vi "TweezerTron.vi"() -> ()   [LabVIEW 2020]
uses:
  _Controls/PIFOC Position.ctl
  _Controls/Confocal Controls.ctl
  _Controls/iFlex.ctl
  _Controls/Manlight Controls.ctl
  _Controls/Exp Params.ctl
  _Controls/Image Thresholds.ctl
  _Controls/Spots.ctl
  _Controls/Tweezertron Ctrl Refs.ctl
  _Controls/Review Ctrl Refs.ctl
  _Controls/Timer actions.ctl
  <vilib>/Platform/TimedLoop/XDataNode/timing_clust.ctl
  <vilib>/Platform/TimedLoop/XDataNode/nitl_modes.ctl
  <vilib>/Platform/TimedLoop/XDataNode/wakeup.ctl
  _Controls/Logging Queue Cluster.ctl
  _Globals/Global Controls.vi
  Instruments/Physik Instrumente/SDK/GCS_LabVIEW_digital/Low Level/Communication.llb/Global1.vi
  <vilib>/Platform/TimedLoop/XDataNode/XDataNode.xnode
  Instruments/Thorlabs/ECU_SDK/ThorECU.lvlib
  Instruments/Thorlabs/LSM_SDK/ThorConfocal.lvlib
  Instruments/Thorlabs/MPH_SDK/MPH16.lvlib
  <vilib>/Platform/TimedLoop/XDataNode/XDNodeRunTimeDep.lvlib
panel:
  out "pane closed":bool
  out "Pause Live Imaging":bool
  out "Live Imaging":bool
  out "Live Review":bool
  out "LiveDisp":T1(plugin-control)
  in  "Control Tabs":T2(tab)
  in  "img thresholds":T3={"Channel A"={1, 16382}, "Channel B"={1, 16382}} {"Channel B" scale=0.0..16382.0; "Channel A" scale=0.0..16382.0}
  in  "Manlight Controls":T4 caption="Trapping Laser" {"Manlight Power" min=0.0 max=10.0 step=0.1 scale=0.0..10.0}
  in  "Stop Live Imaging":bool
  in  "Start Live Imaging":bool
  in  "LSM Settings":T5={"Channel Selection"=enum."A", "Pixel Count"={"Pixels in X"=512, "Pixels in Y"=512}, "Field Size"=90.0, "Frames"=2, "Averaging"=FALSE, "Alignment"=0.0, "Scan Mode"=TRUE, "Gain"={"Gain A"=1, "Gain B"=1}, "Enable PMTs"={"A"=TRUE, "B"=TRUE}, "Voltage Range"={"Range A"=10, "Range B"=10}, "Multi Frame Count"=0.0, "Trigger Mode"=2.0, "Real Time Averaging"=TRUE, "PFOV"=0.0, "MicronsPerPx"=0.0} caption="Confocal Scanner" {"Field Size" min=5.0 max=255.0 step=1.0 scale=5.0..255.0; "PFOV" min=1.0 max=300.0 step=0.1; "MicronsPerPx" min=0.01 step=0.01 format="%.2f"; "Gain"."Gain B" min=1 max=100 step=1; "Gain"."Gain A" min=1 max=100 step=1; "Voltage Range"."Range B" items=["100mV"=5, "200mV"=6, "400mV"=7, "1V"=10, "2V"=11, "4V"=12]; "Voltage Range"."Range A" items=["100mV"=5, "200mV"=6, "400mV"=7, "1V"=10, "2V"=11, "4V"=12]; "Pixel Count"."Pixels in Y" items=["32"=32, "64"=64, "128"=128, "256"=256, "512"=512, "1024"=1024, "2048"=2048]; "Pixel Count"."Pixels in X" items=["32"=32, "64"=64, "128"=128, "256"=256, "512"=512, "1024"=1024, "2048"=2048]}
  in  "PIFOC Settings":T6={"PIFOC Position (mm) [SET]"=0.0, "PIFOC Position\n(um) [ACT]"=0.0087, "last command"=""} {"PIFOC Position\n(um) [ACT]" format="%.2f"; "PIFOC Position (mm) [SET]" min=0.0 max=100.0 step=0.1 scale=0.0..100.0}
  out "LSM Frame Rate":dbl=15.255953524835265 caption="Frame Rate (Hz)" format="%#.0f"
  in  "iFlex Control":T7 caption="Confocal Laser" {"561" min=12.5 max=100.0 step=0.1 scale=0.0..100.0; "488" min=30.0 max=100.0 step=0.1 scale=0.0..100.0}
  in  "PinSelector":dbl(ring)=6.0 caption="Pin Hole (mm)" items=["25", "30", "35", "40", "45", "50", "60", "70", "80", "90", "100", "125", "200", "300", "1000", "2000"]
  in  "Spots":T8=[{"Intensity"=1.0, "Vortex"=0.0, "Phase"=0.0, "X"=7.0, "Y"=0.0, "Z"=0.0}] {"Z" format="%_4g"; "Y" format="%_4g"; "X" format="%_4g"; "Phase" format="%_4g"; "Intensity" format="%_4g"}
  out "Saving To Disk":i32(slide) scale=0.0..8000.0
  out "Acquiring Data":i32(slide) max=1000 scale=0.0..8000.0
  in  "Stop Experiment":bool
  in  "Exp Params":T9={"Experiment Type"="2D Snapshot", "Experiment Name"="Experiment_1", "ExpPath"=path "E:/Data", "TSFrames"=1000, "TSfps"=1000, "ZTSFrames"=1000, "ZTSdt"=1, "Streaming"=FALSE, "Z Stack Settings"={"Start"=0.0, "Step Size"=0.1, "Finish"=1.0}, "total images"=1, "tdms ref"=refnum, "frame #"=0, "images per stack"=1, "total stacks"=1, "period"=1, "PI MVR Increment"=""} {"period" min=1; "total stacks" min=1; "images per stack" min=1; "total images" min=1; "Z Stack Settings"."Start" min=0.0 max=100.0 step=0.1; "Z Stack Settings"."Step Size" min=0.1 max=100.0 step=0.1; "Z Stack Settings"."Finish" min=0.0 max=100.0 step=0.1; "TSFrames" min=1 step=1; "ZTSdt" min=1 step=1; "ZTSFrames" min=2 step=1; "TSfps" min=1 max=1000 step=1}
  in  "Start Experiment":bool
  out "#stack":i32 caption="Stacks"
  in  "Rev Path":path=path "D:/Data/test/qwerty6/qwerty6.tdms" caption="Path to Experiment TDMS File"
  out "dts (ms)":u64[](graph)
  in  "RevFrame":i32(slide)=1 caption="Frame" min=1 max=8001 step=1 scale=0.9..8001.0
  out "Time (s)":dbl
  out "Position (um)":dbl=49.99
  out "dt (ms)":u32
  in  "End Review":bool
  out "PIFOC Positions":cluster{dbl[], "PI pos (um)":dbl[]}(graph)
  in  "Review Experiment":bool
  in  "Save TIFFs":bool
  out "Exporting TIFFS":i32(slide) max=1000 scale=0.0..8000.0
  out "status":string="Status"
  in  "Master Stop":bool
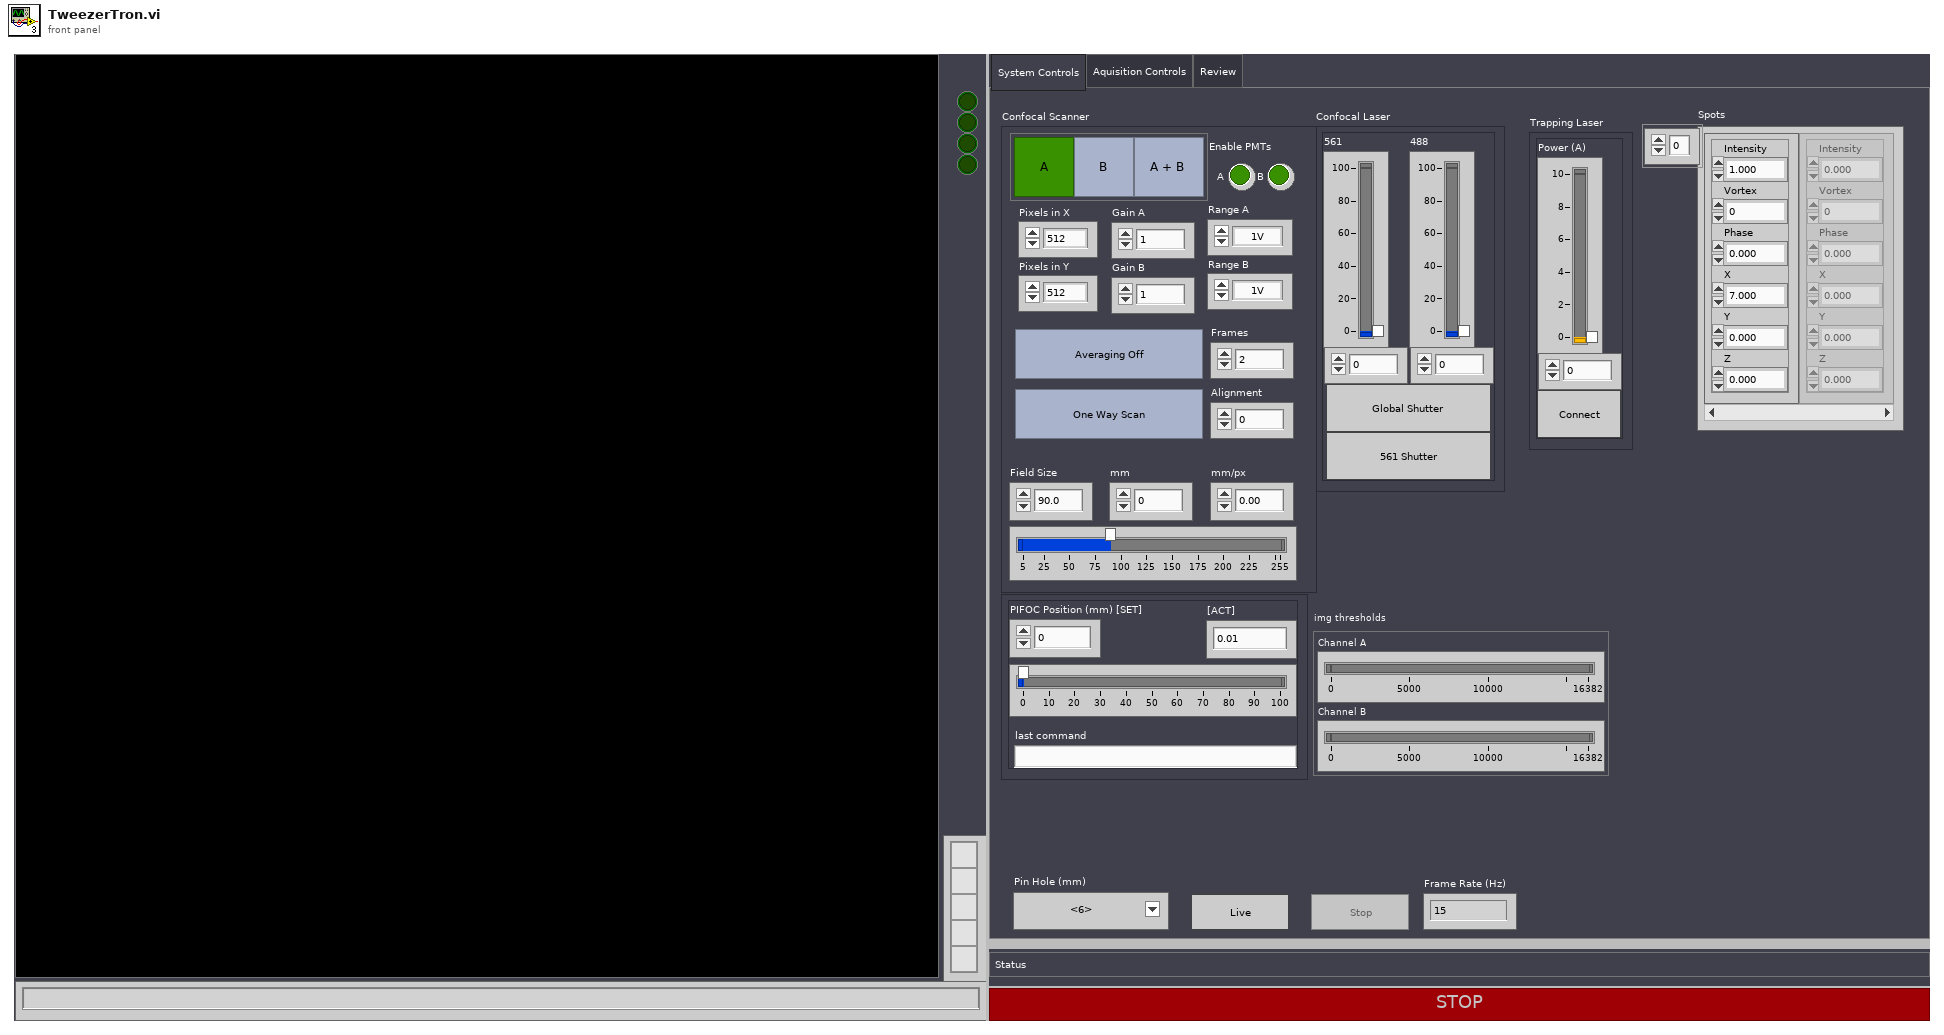
[diagram p1: front panel]
types:
  T1 = typedef "IMAQ Image.ctl" = refnum<image>
  T2 = enum32{"System Controls", "Aquisition Controls", "Review"}
  T3 = typedef "Image Thresholds.ctl" = cluster{"Channel A":cluster{u16, u16}, "Channel B":cluster{u16, u16}}
  T4 = typedef "Manlight Controls.ctl" = cluster{"Manlight Power":dbl, "Open Serial":bool, "VISA Refnum":refnum<visa-resource-name>}
  T5 = typedef "Confocal Controls.ctl" = cluster{"Channel Selection":enum32{"A", "B", "AB"}, "Pixel Count":cluster{"Pixels in X":u32, "Pixels in Y":u32}, "Field Size":dbl, "Frames":u8, "Averaging":bool, "Alignment":dbl, "Scan Mode":bool, "Gain":cluster{"Gain A":u8, "Gain B":u8}, "Enable PMTs":cluster{"A":bool, "B":bool}, "Voltage Range":cluster{"Range A":u16, "Range B":u16}, "Multi Frame Count":dbl, "Trigger Mode":dbl, "Real Time Averaging":bool, "PFOV":dbl, "MicronsPerPx":dbl}
  T6 = typedef "PIFOC Position.ctl" = cluster{"PIFOC Position (mm) [SET]":dbl, "PIFOC Position\n(um) [ACT]":dbl, "last command":string}
  T7 = typedef "iFlex.ctl" = cluster{"561":dbl, "488":dbl, "Global Shutter":bool, "561 Shutter":bool}
  T8 = typedef "Spots.ctl" = cluster{"Intensity":dbl, "Vortex":dbl, "Phase":dbl, "X":dbl, "Y":dbl, "Z":dbl}[]
  T9 = typedef "Exp Params.ctl" = cluster{"Experiment Type":string, "Experiment Name":string, "ExpPath":path, "TSFrames":i32, "TSfps":i32, "ZTSFrames":i32, "ZTSdt":i32, "Streaming":bool, "Z Stack Settings":cluster{"Start":dbl, "Step Size":dbl, "Finish":dbl}, "total images":i32, "tdms ref":refnum<k34>, "frame #":i64, "images per stack":i32, "total stacks":i32, "period":i32, "PI MVR Increment":string}
  T10 = typedef "Image Type" = u32
  T11 = typedef "Review Ctrl Refs.ctl" = cluster{"RevFrame":refnum<vi>, "dts (ms)":refnum<vi>, "PIFOC Positions":refnum<vi>}
  T12 = enum8{"Enabled", "Disabled", "Disabled and Grayed Out"}
  T13 = typedef "Tweezertron Ctrl Refs.ctl" = cluster{"LSM Settings":refnum<vi>, "iFlex Control":refnum<vi>, "PIFOC Settings":refnum<vi>, "PinSelector":refnum<vi>, "Manlight Controls":refnum<vi>, "Exp Params":refnum<vi>, "Image Thresholds":refnum<vi>, "RevFrame":refnum<vi>, "Spots":refnum<vi>}
  T14 = cluster{"Confocal":bool, "Pinhole":bool, "PIFOC":bool, "Manlight":bool, "iFlex":bool, "SLM":bool}
  T15 = typedef "All Controls For Saving.ctl" = cluster{"Confocal Controls":T5, "iFlex Control":T7, "PIFOC Settings":T6, "PinSelector":dbl, "Manlight Controls":T4, "Exp Params":T9, "Spots":T8}
  T16 = typedef "Notifiers.ctl" = cluster{"Instrument Control":refnum<notifier>, "LSM Run Live":refnum<notifier>, "LSM Run Exp":refnum<notifier>, "Review Exp":refnum<notifier>}
  T17 = typedef "Timer actions.ctl" = enum16{"Reset", "Snap", "Total"}
  T18 = cluster{"notification":string, "Variant":variant}
  T19 = cluster{"561":bool, "488":bool, "Global Shutter":bool, "561 Shutter":bool}
  T20 = cluster{"New LSM Settings":T5, "index of change":i32}
  T21 = cluster{"iFlex Controls":T7, "appended array":i32[]}
  T22 = cluster{"Experiment Type":string, "Variant":variant}
  T23 = typedef "XDNodeRunTimeDep.lvlib/timing_clust.ctl" = cluster{"Expected End [f-1]":u64, "Actual End [f-1]":u64, "Finished Late? [f-1]":bool, "Expected End [i-1]":u64, "Actual End [i-1]":u64, "Finished Late? [i-1]":bool, "Expected Start [i]":u64, "Actual Start [i]":u64, "Expected Start [f]":u64, "Actual Start [f]":u64, "Source Name":string, "Structure Name":string, "Period":i64, "Deadline":i64, "Offset":i64, "Start":i64, "Priority":i32, "Timeout":i32, "Mode":T24, "Wakeup Reason":T25, "Error":errorcluster, "Source Type":string, "Secondary Source Type":string, "Global End Time":u64, "Global Start Time":u64, "Frame Duration":u64, "Iteration Duration":u64, "Assigned CPU":i32, "I/O Scan Engine Mode":u32}
  T24 = typedef "XDNodeRunTimeDep.lvlib/nitl_modes.ctl" = enum32{"No Change", "Process missed periods, maintain original phase", "Discard missed periods, maintain original phase", "Process missed periods, ignore original phase", "Discard missed periods, ignore original phase"}
  T25 = typedef "XDNodeRunTimeDep.lvlib/wakeup.ctl" = enum32{"Normal", "Aborted", "Asynchronous wakeup", "Timing source error", "Timed loop error", "Timeout"}
  T26 = typedef "Logging Queue Cluster.ctl" = cluster{"message":string, "Data for Logging":cluster{"pDataBuffer":u16[], "timestamp (ns)":u64, "PI pos (um)":dbl}, "Tweezertron Ctrl Refs":T13}
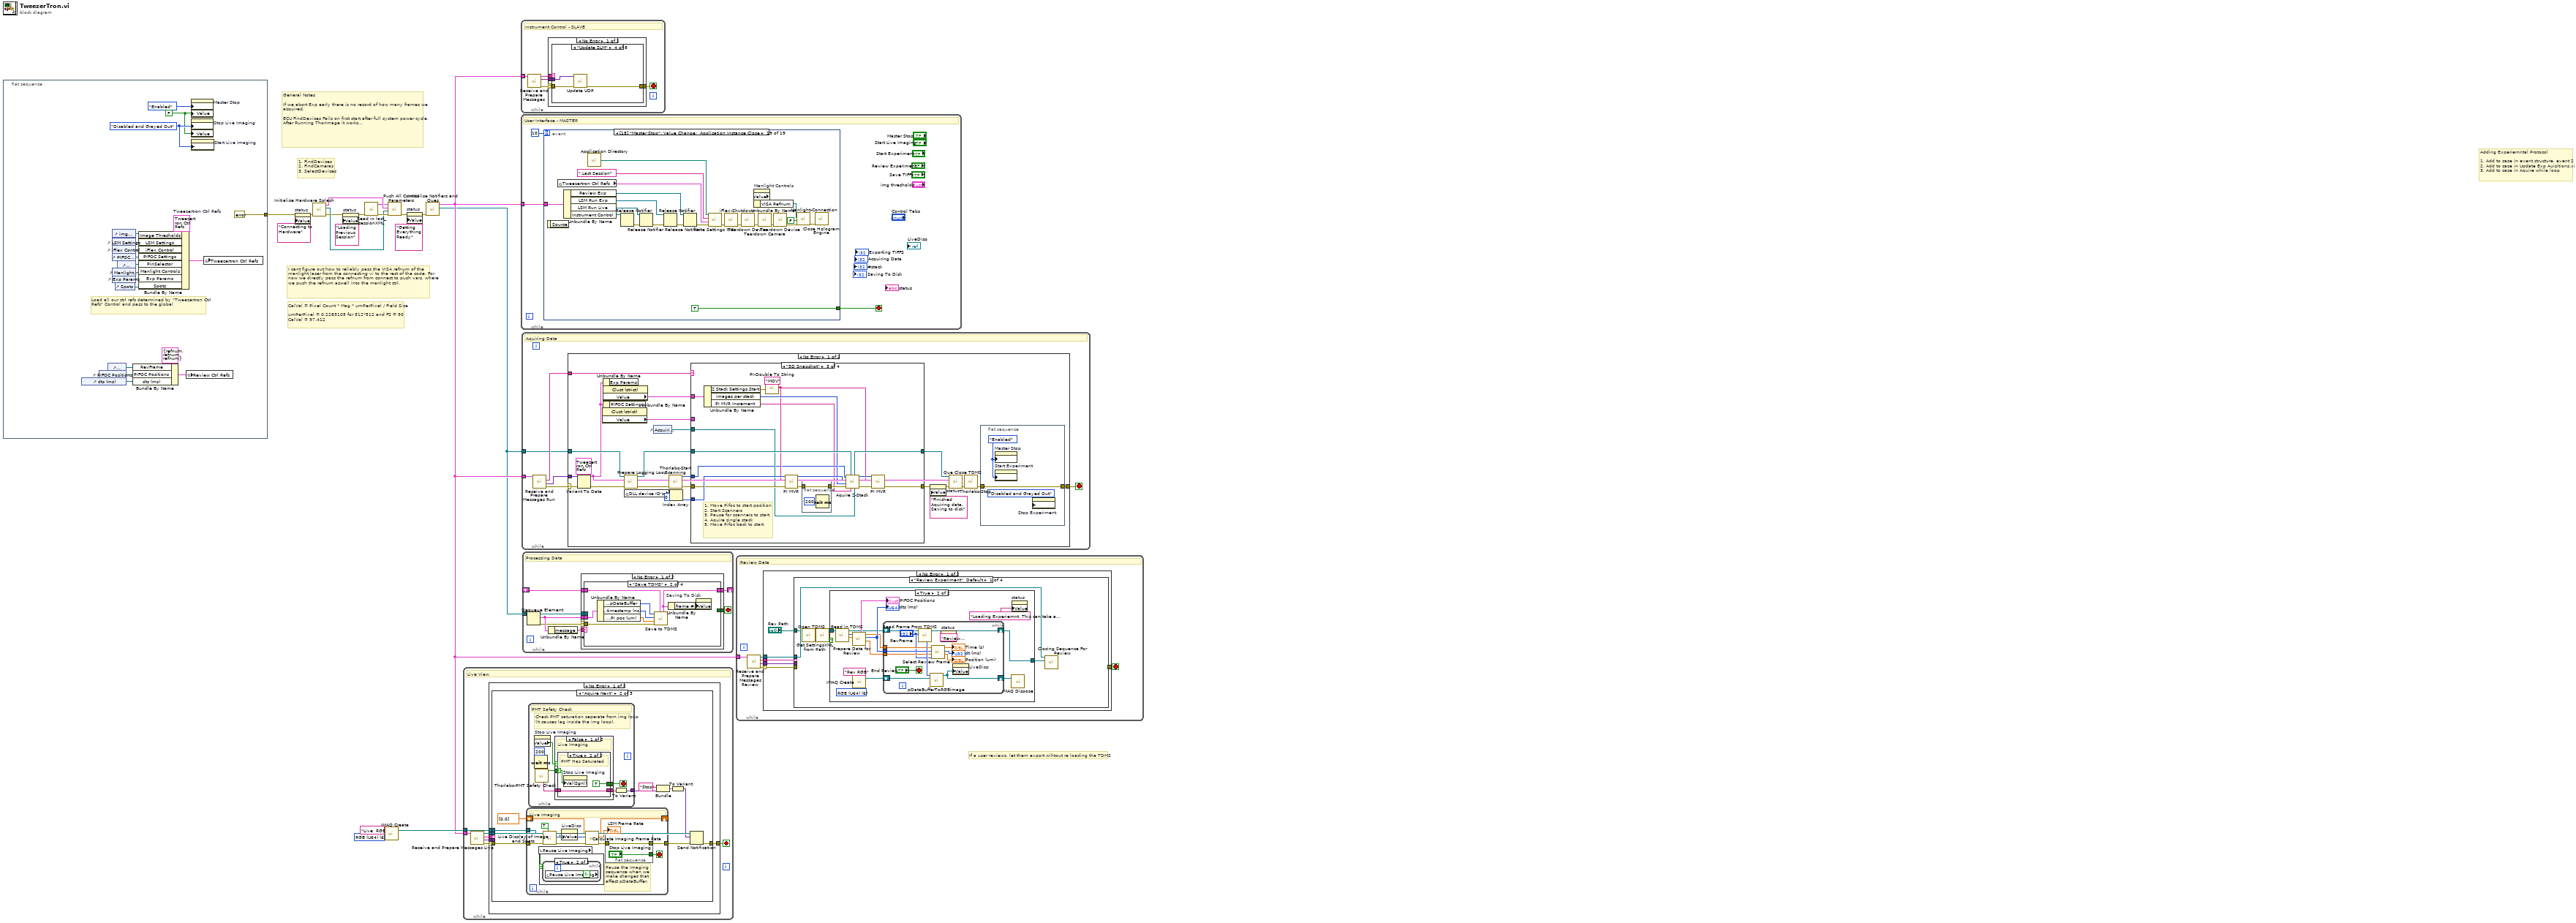
[diagram p0: block diagram]
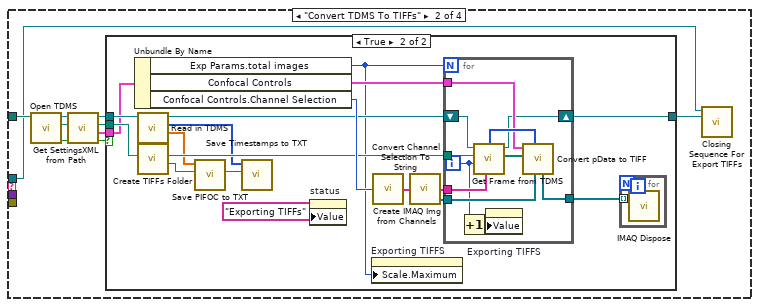
[diagram p3: hidden frame]
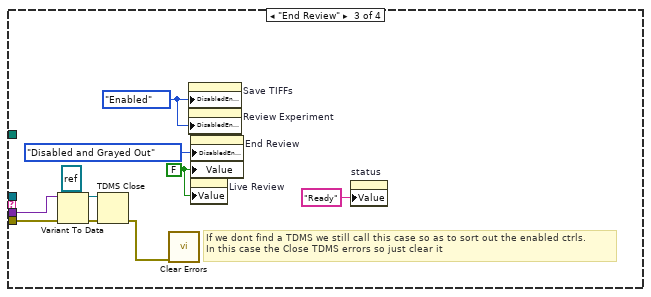
[diagram p5: hidden frame]
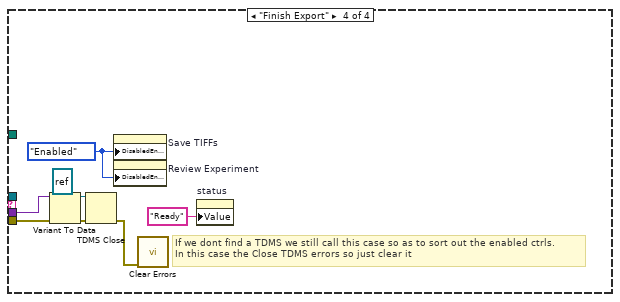
[diagram p6: hidden frame]
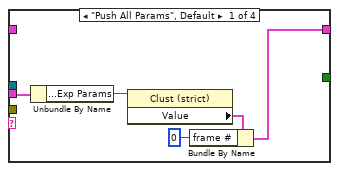
[diagram p8: hidden frame]
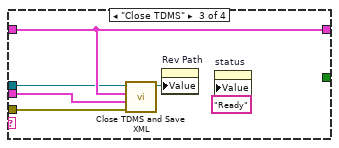
[diagram p9: hidden frame]
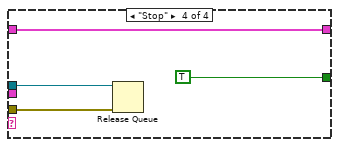
[diagram p10: hidden frame]
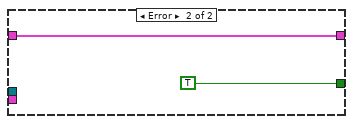
[diagram p11: hidden frame]
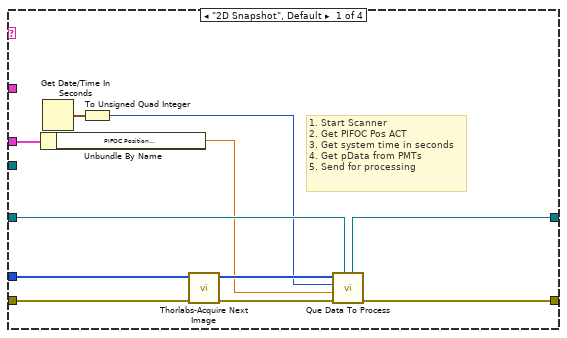
[diagram p12: hidden frame]
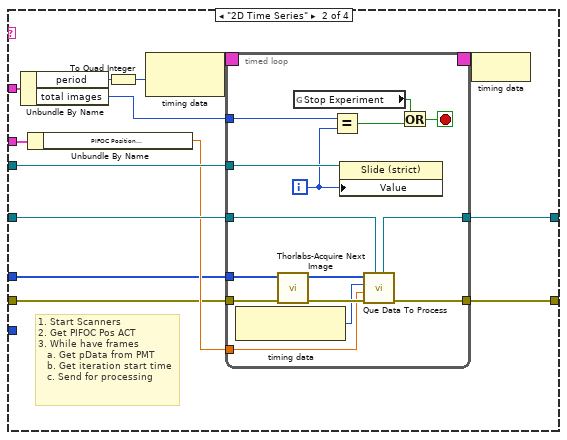
[diagram p13: hidden frame]
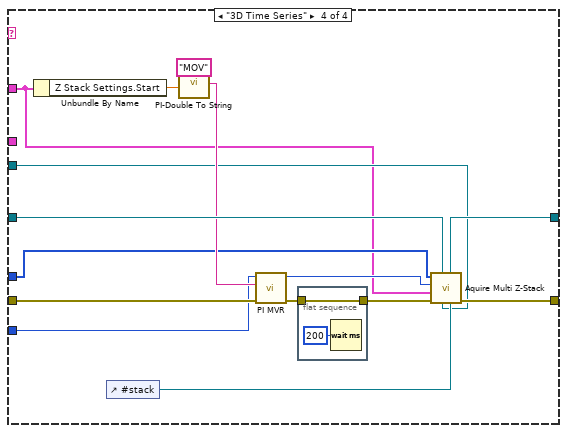
[diagram p14: hidden frame]
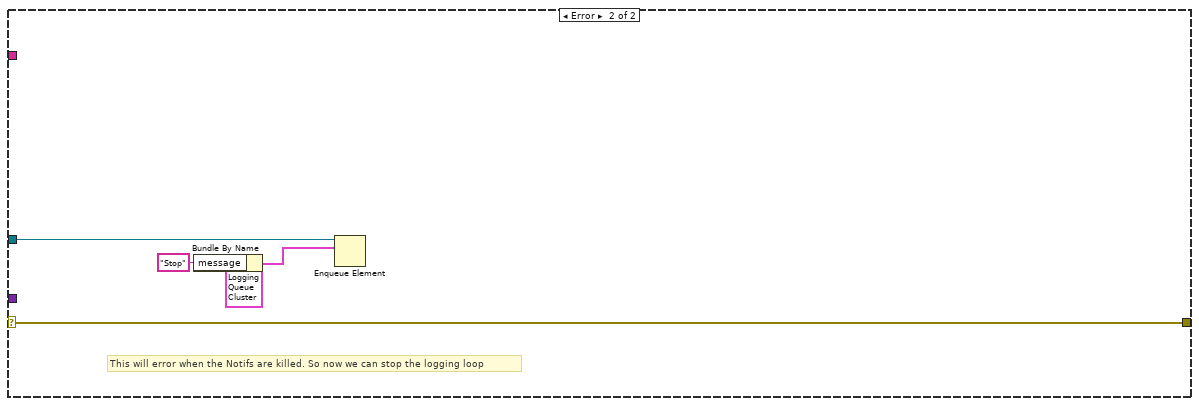
[diagram p15: hidden frame]
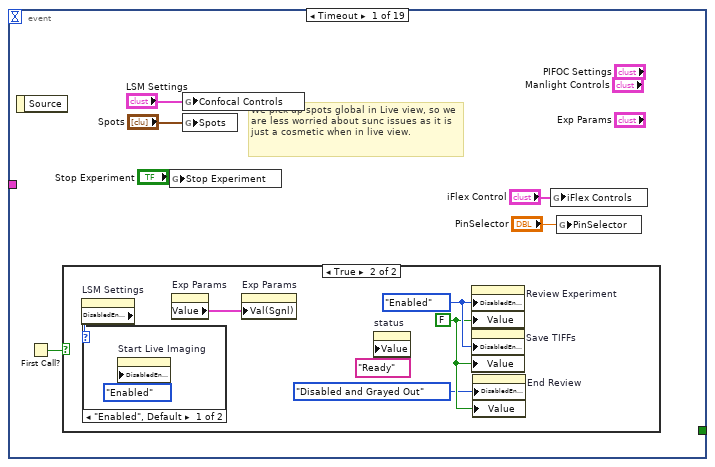
[diagram p16: hidden frame]
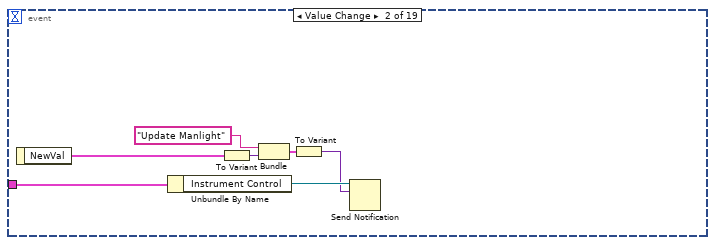
[diagram p19: hidden frame]
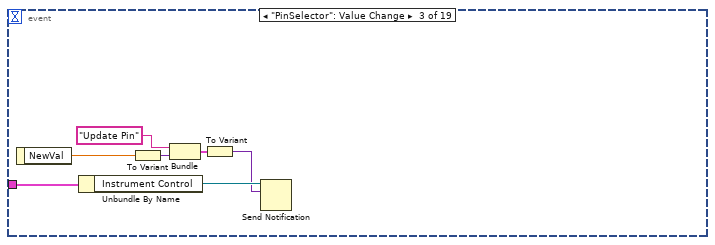
[diagram p20: hidden frame]
diagram:
  w15 = T10 6 items=["Grayscale (U8)", "Grayscale (I16)", "Grayscale (SGL)", "Complex (CSG)", "RGB (U32)", "HSL (U32)", "RGB (U64)", "Grayscale (U16)"] ("Image Type")
  # "If a user reviews, let them export wihtout re loading the TDMS"
  # "General Notes\n\nIf we abort Exp early there is no record of how many frames we acquired.\n\nECU FindDevices Fails on first start after full system power cycle. After Running ThorImage it works..."
  # "Adding Experiemntal Protocol\n\n1. Add to case in event structure, event 2\n2. Add to case in Update Exp Auisitions.vi\n3. Add to case in Aquire while loop"
  # "I cant figure out how to reliably pass the VISA refnum of the manlight laser from the connecting vi to the rest of the code. For now we directly pass the refnum from connect to push vars, where we push the refnum aswell into the manlight ctrl."
  # "CalVal = Pixel Count * Mag * umPerPixel / Field Size\n\numPerPixel = 0.2283105 for 512*512 and FS = 90\nCalVal = 97.412"
  # "1. FindDevices\n2. FindCameras\n3. SelectDevices"
  n1 = flat-sequence {
    tunnel: [errorcluster {"status"=FALSE, "code"=0, "source"=""} ("error constant")] -> w12
    frame #0 {
      w26 = FALSE ("Master Stop")
      w30 = T13 {"LSM Settings"=refnum, "iFlex Control"=refnum, "PIFOC Settings"=refnum, "PinSelector"=refnum, "Manlight Controls"=refnum, "Exp Params"=refnum, "Image Thresholds"=refnum, "RevFrame"=refnum, "Spots"=refnum}  # Tweezertron Ctrl Refs
      w28 = T12."Disabled and Grayed Out" ("Disabled")
      # "Load all our ctrl refs determined by \"Tweezertron Ctrl Refs\" Control and pass to the global"
      n2 = control-ref of="dts (ms)"() -> (w22:refnum<vi>)
      n3 = control-ref of="PIFOC Positions"() -> (w19:refnum<vi>)
      n4 = control-ref of="RevFrame"() -> (w23:refnum<vi>)
      n5 = control-ref of="img thresholds"() -> (w25:refnum<vi>)
      n6 = control-ref of="LSM Settings"() -> (w31:refnum<vi>)
      n7 = control-ref of="iFlex Control"() -> (w35:refnum<vi>)
      n8 = control-ref of="PIFOC Settings"() -> (w34:refnum<vi>)
      n9 = control-ref of="Manlight Controls"() -> (w29:refnum<vi>)
      n10 = control-ref of="Exp Params"() -> (w27:refnum<vi>)
      n11 = control-ref of="Spots"() -> (w20:refnum<vi>)
      n12 = control-ref of="PinSelector"() -> (w32:refnum<vi>)
      n13 = Bundle By Name(cluster=T11 {"RevFrame"=refnum, "dts (ms)"=refnum, "PIFOC Positions"=refnum} ("Review Ctrl Refs"), "RevFrame"=w23, "PIFOC Positions"=w19, "dts (ms)"=w22) -> (w21:T11)
      n14 = Bundle By Name(cluster=w30, "Image Thresholds"=w25, "LSM Settings"=w31, "iFlex Control"=w35, "PIFOC Settings"=w34, "PinSelector"=w32, "Manlight Controls"=w29, "Exp Params"=w27, "Spots"=w20) -> (w33:T13)
      n15 = global write "Global Controls.vi" "Review Ctrl Refs"(w21) -> ()
      n16 = property on="Master Stop" class="Bool (strict)"("DisabledEnum"=T12."Enabled" ("Disabled"), "Value"=w26) -> ()  [unwired: 2 in, 2 out]
      n17 = property on="Stop Live Imaging" class="Bool (strict)"("DisabledEnum"=w28, "Value"=w26) -> ()  [unwired: 2 in, 2 out]
      n18 = property on="Start Live Imaging" class="Bool"("DisabledEnum"=w28) -> ()  [unwired: 2 in, 2 out]
      n19 = global write "Global Controls.vi" "Tweezertron Ctrl Refs"(w33) -> ()
    }
  }
  n20 = property on="status" class="Str"(error in=w12, "Value"="Connecting to Hardware" ("status")) -> (error out=w17:errorcluster)  [unwired: 1 in, 1 out]
  n21 = call "Initialise Hardware Splash.vi"("error in (no error)"=w17) -> ("error out"=w1:errorcluster, "VISA Refnum out"=w5:refnum<visa-resource-name>, "Enabled Hardware"=w11:T14)  [unwired: 8 in]
  n22 = property on="status" class="Str"(error in=w1, "Value"="Loading Previous Session" ("status")) -> (error out=w14:errorcluster)  [unwired: 1 in, 1 out]
  n23 = call "Read in last_sessionXML.vi"("error in"=w14) -> ("error out"=w8:errorcluster, "All Controlls For Saving"=w9:T15)  [unwired: 9 in]
  n24 = call "IMAQ Create"("Image Name"="Live  RGB", "Image Type"=w15) -> ("New Image"=w4:T1)  [unwired: 3 in, 1 out]
  n25 = call "Push All Control Parameters.vi"("error in"=w8, "Manlight VISA Refnum"=w5, "Enabled Hardware"=w11, "All Controlls For Savinge"=w9) -> ("error out"=w6:errorcluster)  [unwired: 5 in]
  n26 = property on="status" class="Str"(error in=w6, "Value"="Getting Everything Ready" ("status")) -> (error out=w10:errorcluster)  [unwired: 1 in, 1 out]
  n27 = call "Initialise Notifiers and Ques.vi"("error in (no error)"=w10) -> ("Logging Queue out"=w2:refnum<queue>, "Notifiers"=w3:T16)  [unwired: 8 in, 1 out]
  n28 = while {
    tunnel: w4 -> [w44]
    tunnel: w3 -> [w38]
    stop <- w41 stop-if-true
    # "Live View"
    n29 = call "Receive and Prepare Messages Live.vi"("Notifiers"=w38) -> ("error out"=w42:errorcluster, "params"=w39:variant, "message"=w40:string, "LSM Run Live"=w43:refnum<notifier>)  [unwired: 6 in]
    n30 = case shown="No Error" w42 {
      selector: w42 -> [w49 w117]
      tunnel: w40 -> [w50 _]
      tunnel: w43 -> [w48 _]
      tunnel: w44 -> [w47 _]
      tunnel: [w46 w117] -> w41
      tunnel: w39 -> [w45 _]
      frame No Error {
        n31 = case shown="\"Aquire Next\"" w50 {
          tunnel: w49 -> [w61 w62 w115]
          tunnel: w48 -> [w55 w69 _]
          tunnel: w47 -> [_ w71 _]
          tunnel: [w54 w67 w114] -> w46
          tunnel: w45 -> [w53 _ w112]
          frame "Start" {
            n32 = global read "Global Controls.vi" "Tweezertron Ctrl Refs"() -> (w51:T13)
            n33 = Bundle("notification"="Aquire Next", "params"=w53) -> (w57:cluster{"notification":string, "params":variant})  [unwired: 1 in]
            n34 = call "Thorlabs-Start Scanning.vi"("error in (no error)"=w61, "Tweezertron Ctrl Refs"=w51) -> ("error out"=w60:errorcluster)  [unwired: 7 in, 2 out]
            n35 = To Variant(anything=w57) -> (Variant=w56:variant)
            n36 = Send Notification(notification=w56, notifier=w55, error in (no error)=w60) -> (error out=w59:errorcluster)  [unwired: 1 out]
            n37 = call "Get Kernel Time.vi"("error in (no error) in"=w59, "Action (Snap)"=Timer_actions."Reset") -> ("error out"=w54:errorcluster)  [unwired: 8 in, 1 out]
          }
          frame "Aquire Next" {
            n38 = while {
              tunnel: w71 -> [w97]
              tunnel: w62 -> [w102]
              tunnel: [w93] -> w70
              shift-right: [w101] -> _
              shift-left: dbl[] [0.0] -> [w95]
              stop <- w92 stop-if-true
              # "Pause the Imaging sequence when we make changes that affect pDataBuffer."
              # "Live Imaging"
              n39 = local read "Pause Live Imaging"() -> (w96:bool)
              n40 = case shown="True" w96 {
                frame False {
                }
                frame True {
                  n41 = while {
                    stop <- w105 continue-if-true
                    n42 = local read "Pause Live Imaging"() -> (w105:bool)
                  }
                }
              }
              n43 = call "Live Display of Image and Spots.vi"("Draw spots"=TRUE, "error in (no error)"=w102, "img dst"=w97) -> ("error out"=w98:errorcluster, "Frame Duration"=w100:i64, "img out"=w91:refnum<image>)  [unwired: 6 in]
              n44 = property on="LiveDisp" class="ImageControl"("Value"=w91) -> ()  [unwired: 2 in, 2 out]
              n45 = call "Calculate Imaging Frame Rate.vi"("error in (no error)"=w98, "Frame Duration"=w100, "Durations IN"=w95) -> ("error out"=w94:errorcluster, "LSM Frame Rate"=→"LSM Frame Rate":dbl, "Durations OUT"=w101:dbl[])  [unwired: 6 in]
              n46 = flat-sequence {
                tunnel: w94 -> [w104]
                tunnel: [w104] -> w93
                tunnel: ["Stop Live Imaging"] -> w92
                frame #0 {
                }
              }
            }
            n47 = while {
              tunnel: [w73] -> w63
              stop <- w72 stop-if-true
              # "Check PMT saturation seperate from img loop (It causes lag inside the img loop)."
              # "PMT Safety Check"
              n48 = property on="Stop Live Imaging" class="Bool (strict)"() -> ("Value"=w78:bool)  [unwired: 2 in, 2 out]
              n49 = Wait (ms)(milliseconds to wait=u32 200) -> ()  [unwired: 1 out]
              n50 = call "Thorlabs-PMT Safety Check.vi"() -> ("Stop"=w77:bool, "User message"=w75:string)  [unwired: 9 in, 1 out]
              n51 = case shown="False" w78 {
                selector: w78 -> [_ w89]
                tunnel: [w81 w89] -> w72
                tunnel: w77 -> [w82 _]
                tunnel: w75 -> [w80 _]
                tunnel: [w79 "" ("User message")] -> w74
                frame False {
                  # "Live Imaging"
                  n52 = case shown="True" w82 {
                    selector: w82 -> [w84 w87]
                    tunnel: [w84 TRUE] -> w81
                    tunnel: w80 -> [_ w85]
                    tunnel: ["" ("User message") w85] -> w79
                    frame False {
                      # "All Good"
                    }
                    frame True {
                      # "PMT Has Saturated"
                      n53 = property on="Stop Live Imaging" class="Bool (strict)"("Val(Sgnl)"=w87) -> ()  [unwired: 2 in, 2 out]
                    }
                  }
                }
                frame True {
                  # "Stop"
                }
              }
              n54 = To Variant(anything=w74) -> (Variant=w73:variant)
            }
            n55 = Bundle("notification"="Stop", "Variant"=w63) -> (w66:T18)  [unwired: 1 in]
            n56 = To Variant(anything=w66) -> (Variant=w64:variant)
            n57 = Send Notification(notification=w64, notifier=w69, error in (no error)=w70) -> (error out=w67:errorcluster)  [unwired: 1 out]
          }
          frame "Stop", Default {
            w108 = T12."Enabled" ("Disabled")
            # "If we sent the stop message because the PMTs saturated, let the user know"
            n58 = Variant To Data(type="", Variant=w112) -> (data=w109:string)  [unwired: 1 in, 1 out]
            n59 = Empty String/Path?(string/path=w109) -> (empty?=w110:bool)
            n60 = case shown="False" w110 {
              tunnel: w109 -> [w116 _]
              frame False {
                n61 = call "Display Message to User"("Message"=w116) -> ()  [unwired: 9 in, 2 out]
              }
              frame True {
              }
            }
            n62 = property on="Stop Live Imaging" class="Bool (strict)"("Value"=FALSE ("Stop Live Imaging"), "DisabledEnum"=T12."Disabled and Grayed Out" ("Disabled")) -> ()  [unwired: 2 in, 2 out]
            n63 = call "Thorlabs-Stop.vi"("error in (no error)"=w115) -> ("error out"=w114:errorcluster)  [unwired: 10 in]
            n64 = property on="status" class="Str"("Value"="Ready" ("status")) -> ()  [unwired: 2 in, 2 out]
            n65 = property on="Master Stop" class="Bool (strict)"("DisabledEnum"=w108) -> ()  [unwired: 2 in, 2 out]
            n66 = property on="Start Live Imaging" class="Bool"("DisabledEnum"=w108) -> ()  [unwired: 2 in, 2 out]
          }
        }
      }
      frame Error {
      }
    }
  }
  n67 = while {
    tunnel: w3 -> [w119]
    stop <- w118 stop-if-true
    # "User Interface - MASTER"
    n68 = event shown="[18] \"Master Stop\": Value Change;  Application Instance Close" {
      selector: _ -> [_ _ _ _ _ _ _ _ _ _ _ _ _ _ _ _ _ _ _]
      dyn-events: _ -> [_ _ _ _ _ _ _ _ _ _ _ _ _ _ _ _ _ _ _]
      timeout: 10 -> [_ _ _ _ _ _ _ _ _ _ _ _ _ _ _ _ _ _ _]
      tunnel: w119 -> [_ w135 w142 w157 w162 w172 w182 w191 _ _ w275 w291 w310 w322 _ w331 _ _ w363]
      tunnel: [_ _ _ _ _ _ _ _ _ _ _ _ _ _ _ _ _ _ TRUE] -> w118
      event Timeout {
        # "We pick up spots global in Live view, so we are less worried about sunc issues as it is just a cosmetic when in live view."
        n69 = event-data() -> ()  [unwired: 1 in, 1 out]
        n70 = First Call?() -> (First Call?: T/F=w125:bool)
        n71 = case shown="True" w125 {
          frame False {
          }
          frame True {
            w129 = FALSE ("Review Experiment")
            w130 = T12."Enabled" ("Disabled")
            n72 = property on="LSM Settings" class="Clust (strict)"() -> ("DisabledEnum"=w131:T12)  [unwired: 2 in, 2 out]
            n73 = case shown="\"Enabled\", Default" w131 {
              frame "Enabled", Default {
                n74 = property on="Start Live Imaging" class="Bool"("DisabledEnum"=T12."Enabled" ("Disabled")) -> ()  [unwired: 2 in, 2 out]
              }
              frame "Disabled" {
              }
            }
            n75 = property on="Exp Params" class="Clust (strict)"() -> ("Value"=w127:T9)  [unwired: 2 in, 2 out]
            n76 = property on="Exp Params" class="Clust (strict)"("Val(Sgnl)"=w127) -> ()  [unwired: 2 in, 2 out]
            n77 = property on="status" class="Str"("Value"="Ready" ("status")) -> ()  [unwired: 2 in, 2 out]
            n78 = property on="Review Experiment" class="Bool (strict)"("DisabledEnum"=w130, "Value"=w129) -> ()  [unwired: 2 in, 2 out]
            n79 = property on="Save TIFFs" class="Bool (strict)"("DisabledEnum"=w130, "Value"=w129) -> ()  [unwired: 2 in, 2 out]
            n80 = property on="End Review" class="Bool (strict)"("DisabledEnum"=T12."Disabled and Grayed Out" ("Disabled"), "Value"=w129) -> ()  [unwired: 2 in, 2 out]
          }
        }
        n81 = global write "Global Controls.vi" "Stop Experiment"("Stop Experiment") -> ()
        n82 = global write "Global Controls.vi" "Confocal Controls"("LSM Settings") -> ()
        n83 = global write "Global Controls.vi" "Spots"("Spots") -> ()
        n84 = global write "Global Controls.vi" "iFlex Controls"("iFlex Control") -> ()
        n85 = global write "Global Controls.vi" "PinSelector"("PinSelector") -> ()
      }
      event Value Change {
        n86 = event-data() -> ("NewVal"=w134:T4)  [unwired: 1 in]
        n87 = Unbundle By Name(w135) -> ("Instrument Control"=w140:refnum<notifier>)
        n88 = To Variant(anything=w134) -> (Variant=w136:variant)
        n89 = Bundle("notification"="Update Manlight", "Variant"=w136) -> (w138:T18)  [unwired: 1 in]
        n90 = To Variant(anything=w138) -> (Variant=w137:variant)
        n91 = Send Notification(notification=w137, notifier=w140) -> ()  [unwired: 1 in, 2 out]
      }
      event "PinSelector": Value Change {
        n92 = event-data() -> ("NewVal"=w141:dbl)  [unwired: 1 in]
        n93 = Unbundle By Name(w142) -> ("Instrument Control"=w147:refnum<notifier>)
        n94 = To Variant(anything=w141) -> (Variant=w143:variant)
        n95 = Bundle("notification"="Update Pin", "Variant"=w143) -> (w145:T18)  [unwired: 1 in]
        n96 = To Variant(anything=w145) -> (Variant=w144:variant)
        n97 = Send Notification(notification=w144, notifier=w147) -> ()  [unwired: 1 in, 2 out]
      }
      event Value Change {
        n98 = event-data() -> ("NewVal"=w150:T7, "OldVal"=w155:T7)  [unwired: 1 in]
        n99 = Not Equal?(x=w150, y=w155) -> (x != y?=w154:T19)
        n100 = Cluster To Array(cluster=w154) -> (array=w153:bool[])
        n101 = Search 1D Array(1D array=w153, element=TRUE) -> (index of element=w149:i32)  [unwired: 1 in]
        n102 = Build Array(w149) -> (w148:i32[])
        n103 = Unbundle By Name(w157) -> ("Instrument Control"=w161:refnum<notifier>)
        n104 = Bundle("NewVal"=w150, w148) -> (w151:cluster{"NewVal":T7, i32[]})  [unwired: 1 in]
        n105 = To Variant(anything=w151) -> (Variant=w156:variant)
        n106 = Bundle("notification"="Update iFlex", "Variant"=w156) -> (w158:T18)  [unwired: 1 in]
        n107 = To Variant(anything=w158) -> (Variant=w159:variant)
        n108 = Send Notification(notification=w159, notifier=w161) -> ()  [unwired: 1 in, 2 out]
      }
      event Value Change {
        n109 = event-data() -> ("NewVal"=w164:T6)  [unwired: 1 in]
        n110 = Unbundle By Name(w162) -> ("Instrument Control"=w168:refnum<notifier>)
        n111 = To Variant(anything=w164) -> (Variant=w165:variant)
        n112 = Bundle("notification"="Update PIFOC", "Variant"=w165) -> (w163:T18)  [unwired: 1 in]
        n113 = To Variant(anything=w163) -> (Variant=w166:variant)
        n114 = Send Notification(notification=w166, notifier=w168) -> ()  [unwired: 1 in, 2 out]
      }
      event Value Change {
        n115 = event-data() -> ("OldVal"=w178:T5, "NewVal"=w170:T5)  [unwired: 1 in]
        n116 = flat-sequence {
          tunnel: w172 -> [w179]
          tunnel: [w179] -> w171
          frame #0 {
            "Pause Live Imaging" <- TRUE ("Pause")
          }
        }
        n117 = call "Compare Old and New LSM.vi"("New LSM Settings"=w170, "Old LSM Settings"=w178) -> ("LSM Settings with index of change"=w169:T20)  [unwired: 4 in]
        n118 = Unbundle By Name(w171) -> ("Instrument Control"=w177:refnum<notifier>)
        n119 = To Variant(anything=w169) -> (Variant=w174:variant)
        n120 = Bundle("notification"="Update LSM", "Variant"=w174) -> (w173:T18)  [unwired: 1 in]
        n121 = To Variant(anything=w173) -> (Variant=w175:variant)
        n122 = Send Notification(notification=w175, notifier=w177) -> ()  [unwired: 1 in, 2 out]
      }
      event Value Change {
        n123 = event-data() -> ("NewVal"=w181:T8)  [unwired: 1 in]
        n124 = Unbundle By Name(w182) -> ("Instrument Control"=w187:refnum<notifier>)
        n125 = To Variant(anything=w181) -> (Variant=w184:variant)
        n126 = Bundle("notification"="Update SLM", "Variant"=w184) -> (w183:T18)  [unwired: 1 in]
        n127 = To Variant(anything=w183) -> (Variant=w185:variant)
        n128 = Send Notification(notification=w185, notifier=w187) -> ()  [unwired: 1 in, 2 out]
      }
      event Value Change {
        n129 = event-data() -> ("NewVal"=w196:cluster{"A":bool, "B":bool})  [unwired: 1 in]
        n130 = control-ref of="Channel Selection"() -> (w193:refnum<vi>)
        n131 = property class="RadioBtnsControl (strict)"(reference=w193) -> ("Controls[]"=w192:refnum<vi>[])  [unwired: 1 in, 2 out]
        n132 = Not(x=w196) -> (.not. x?=w195:cluster{"A":bool, "B":bool})
        n133 = Unbundle By Name(w195) -> ("A"=w188:bool, "B"=w189:bool)
        n134 = Or(x=w188, y=w189) -> (x .or. y?=w194:bool)
        n135 = And(x=w188, y=w189) -> (x .and. y?=w190:bool)
        n136 = case shown="False" w194 {
          tunnel: w188 -> [_ w204]
          tunnel: w192 -> [w197 w203]
          tunnel: w191 -> [_ w201]
          tunnel: w190 -> [_ w202]
          frame False {
            n137 = for {
              tunnel: w197 -> [w199] mode=indexing
              tunnel: T12."Enabled" ("Disabled") -> [w200]
              n138 = property class="Ctl"(reference=w199, "DisabledEnum"=w200) -> ()  [unwired: 1 in, 2 out]
            }
          }
          frame True {
            n139 = case shown="True" w202 {
              tunnel: w204 -> [w215 _]
              tunnel: w203 -> [w205 w233]
              tunnel: w201 -> [w206 _]
              frame False {
                n140 = case shown="False" w215 {
                  tunnel: [0 ("index") 1 ("index")] -> w213
                  frame False {
                  }
                  frame True {
                  }
                }
                n141 = flat-sequence {
                  tunnel: w206 -> [w216]
                  frame #0 {
                    # "Only start this once the case has finished"
                    n142 = global read "Global Controls.vi" "Tweezertron Ctrl Refs"() -> (w227:T13)
                    n143 = local write "Pause Live Imaging"(TRUE ("Pause")) -> ()
                    n144 = Unbundle By Name(w227) -> ("LSM Settings"=w226:refnum<vi>)
                    n145 = property class="Clust (strict)"(reference=w226) -> ("Value"=w225:T5)  [unwired: 1 in, 2 out]
                    n146 = Bundle("Value"=w225, 0) -> (w223:cluster{"Value":T5, i32})  [unwired: 1 in]
                    n147 = Unbundle By Name(w216) -> ("Instrument Control"=w222:refnum<notifier>)
                    n148 = To Variant(anything=w223) -> (Variant=w219:variant)
                    n149 = Bundle("notification"="Update LSM", "Variant"=w219) -> (w218:T18)  [unwired: 1 in]
                    n150 = To Variant(anything=w218) -> (Variant=w220:variant)
                    n151 = Send Notification(notification=w220, notifier=w222) -> ()  [unwired: 1 in, 2 out]
                  }
                }
                n152 = Delete From Array(array=w205, length=1, index=w213) -> (deleted portion=w210:refnum<vi>[], array with subset deleted=w212:refnum<vi>[])
                n153 = Index Array(array=w210) -> (element=w209:refnum<vi>)  [unwired: 1 in]
                n154 = To Variant(anything=TRUE) -> (Variant=w207:variant)
                n155 = for {
                  tunnel: w212 -> [w228] mode=indexing
                  tunnel: T12."Disabled and Grayed Out" ("Disabled") -> [w229]
                  n156 = property class="Ctl"(reference=w228, "DisabledEnum"=w229) -> ()  [unwired: 1 in, 2 out]
                }
                n157 = property class="Ctl"(reference=w209, "Value"=w207) -> ()  [unwired: 1 in, 2 out]
              }
              frame True {
                n158 = property on="Stop Live Imaging" class="Bool (strict)"("Value"=TRUE ("Stop Live Imaging")) -> ()  [unwired: 2 in, 2 out]
                n159 = for {
                  tunnel: w233 -> [w235] mode=indexing
                  tunnel: T12."Disabled and Grayed Out" ("Disabled") -> [w236]
                  n160 = property class="Ctl"(reference=w235, "DisabledEnum"=w236) -> ()  [unwired: 1 in, 2 out]
                }
              }
            }
          }
        }
      }
      event Value Change {
        n161 = event-data() -> ()  [unwired: 1 in, 1 out]
        n162 = property on="Exp Params" class="Clust (strict)"() -> ("Value"=w240:T9)  [unwired: 2 in, 2 out]
        n163 = call "Update Exp Auisitions.vi"("ExpVars"=w240) -> ("ExpVars new #aqu"=w239:T9)  [unwired: 9 in, 1 out]
        n164 = Unbundle By Name(w239) -> ("images per stack"=w238:i32, "total images"=w237:i32)
        n165 = property on="Exp Params" class="Clust (strict)"("Value"=w239) -> ()  [unwired: 2 in, 2 out]
        n166 = property on="Acquiring Data" class="Slide (strict)"("Scale.Maximum"=w238) -> ()  [unwired: 2 in, 2 out]
        n167 = property on="Saving To Disk" class="Slide (strict)"("Scale.Maximum"=w237) -> ()  [unwired: 2 in, 2 out]
      }
      event Value Change {
        # "trigers update of #frames"
        n168 = event-data() -> ()  [unwired: 1 in, 1 out]
        n169 = property on="Streaming" class="Bool (strict)"() -> ("Value"=w242:bool)  [unwired: 2 in, 2 out]
        n170 = property on="Experiment Type" class="CmbBox"() -> ("Value"=w243:string)  [unwired: 2 in, 2 out]
        n171 = property on="TSFrames" class="DigNum (strict)"() -> ("Value"=w241:i32)  [unwired: 2 in, 2 out]
        n172 = case shown="\"2D Snapshot\", Default" w243 {
          tunnel: [w250 w254 w258 w262] -> w249
          tunnel: [w250 w253 w258 w259] -> w247
          tunnel: [w250 w253 w258 w260] -> w246
          tunnel: [w250 w254 w258 w259] -> w245
          tunnel: [w250 w251 w258 w262] -> w248
          tunnel: [w250 w253 TRUE w259] -> w244
          tunnel: w242 -> [_ w252 _ w261]
          frame "2D Snapshot", Default {
            w250 = FALSE
          }
          frame "2D Time Series" {
            w254 = TRUE
            w253 = FALSE
            n173 = case shown="False" w252 {
              tunnel: [TRUE FALSE] -> w251
              frame False {
              }
              frame True {
              }
            }
          }
          frame "3D Snapshot" {
            w258 = FALSE
          }
          frame "3D Time Series" {
            w262 = FALSE
            w259 = TRUE
            n174 = case shown="True" w261 {
              tunnel: [TRUE FALSE] -> w260
              frame False {
              }
              frame True {
              }
            }
          }
        }
        n175 = property on="TSFrames" class="DigNum (strict)"("Val(Sgnl)"=w241) -> ()  [unwired: 2 in, 2 out]
        n176 = property on="TSFrames" class="DigNum (strict)"("Visible"=w249) -> ()  [unwired: 2 in, 2 out]
        n177 = property on="TSfps" class="DigNum (strict)"("Visible"=w248) -> ()  [unwired: 2 in, 2 out]
        n178 = property on="ZTSFrames" class="DigNum (strict)"("Visible"=w247) -> ()  [unwired: 2 in, 2 out]
        n179 = property on="ZTSdt" class="DigNum (strict)"("Visible"=w246) -> ()  [unwired: 2 in, 2 out]
        n180 = property on="Streaming" class="Bool (strict)"("Visible"=w245) -> ()  [unwired: 2 in, 2 out]
        n181 = property on="Z Stack Settings" class="Clust (strict)"("Visible"=w244) -> ()  [unwired: 2 in, 2 out]
      }
      event "Start Live Imaging": Value Change {
        w283 = T12."Disabled and Grayed Out" ("Disabled")
        # "Open iFlex Global Shutter then start scanning"
        n182 = event-data() -> ()  [unwired: 1 in, 1 out]
        n183 = global read "Global Controls.vi" "iFlex Controls"() -> (w270:T7)
        n184 = Bundle By Name(cluster=w270, "Global Shutter"=TRUE) -> (w268:T7)
        n185 = global read "Global Controls.vi" "Tweezertron Ctrl Refs"() -> (w266:T13)
        n186 = property on="iFlex Control" class="Clust (strict)"("Val(Sgnl)"=w268) -> ()  [unwired: 2 in, 2 out]
        n187 = property on="Master Stop" class="Bool (strict)"("DisabledEnum"=w283) -> ()  [unwired: 2 in, 2 out]
        n188 = property on="Start Live Imaging" class="Bool"("DisabledEnum"=w283) -> ()  [unwired: 2 in, 2 out]
        n189 = Unbundle By Name(w275) -> ("LSM Run Live"=w274:refnum<notifier>, "Instrument Control"=w281:refnum<notifier>)
        n190 = Bundle("iFlex Controls"=w268, "appended array"=i32[] [2]) -> (w276:T21)  [unwired: 1 in]
        n191 = To Variant(anything=w276) -> (Variant=w277:variant)
        n192 = Bundle("notification"="Update iFlex", "Variant"=w277) -> (w278:T18)  [unwired: 1 in]
        n193 = To Variant(anything=w278) -> (Variant=w279:variant)
        n194 = Send Notification(notification=w279, notifier=w281) -> (error out=w271:errorcluster)  [unwired: 1 in, 1 out]
        n195 = To Variant(anything=w266) -> (Variant=w267:variant)
        n196 = property on="Stop Live Imaging" class="Bool (strict)"("DisabledEnum"=T12."Enabled" ("Disabled")) -> ()  [unwired: 2 in, 2 out]
        n197 = property on="status" class="Str"("Value"="Scanning" ("status")) -> ()  [unwired: 2 in, 2 out]
        n198 = Bundle("notification"="Start", "Variant"=w267) -> (w284:T18)  [unwired: 1 in]
        n199 = To Variant(anything=w284) -> (Variant=w285:variant)
        n200 = Send Notification(notification=w285, notifier=w274, error in (no error)=w271) -> ()  [unwired: 2 out]
        "Live Imaging" <- TRUE ("Live Imaging")
      }
      event "Stop Live Imaging": Value Change {
        # "Shut iFlex Global Shutter"
        n201 = event-data() -> ()  [unwired: 1 in, 1 out]
        n202 = global read "Global Controls.vi" "iFlex Controls"() -> (w290:T7)
        n203 = Bundle By Name(cluster=w290, "Global Shutter"=FALSE) -> (w288:T7)
        n204 = property on="iFlex Control" class="Clust (strict)"("Val(Sgnl)"=w288) -> ()  [unwired: 2 in, 2 out]
        n205 = Unbundle By Name(w291) -> ("Instrument Control"=w298:refnum<notifier>)
        n206 = Bundle("iFlex Controls"=w288, "appended array"=i32[] [2]) -> (w293:T21)  [unwired: 1 in]
        n207 = To Variant(anything=w293) -> (Variant=w294:variant)
        n208 = Bundle("notification"="Update iFlex", "Variant"=w294) -> (w295:T18)  [unwired: 1 in]
        n209 = To Variant(anything=w295) -> (Variant=w296:variant)
        n210 = property on="Live Imaging" class="Bool (strict)"("Value"=FALSE ("Live Imaging")) -> ()  [unwired: 2 in, 2 out]
        n211 = Send Notification(notification=w296, notifier=w298) -> ()  [unwired: 1 in, 2 out]
      }
      event "Start Experiment": Value Change {
        w304 = T12."Disabled and Grayed Out" ("Disabled")
        # "We should push all current ctrls just to be sure they are up to date"
        # "Open iFlex Global Shutter then start start exp"
        n212 = event-data() -> ()  [unwired: 1 in, 1 out]
        n213 = Unbundle By Name(w310) -> ("LSM Run Exp"=w309:refnum<notifier>, "Instrument Control"=w311:refnum<notifier>)
        n214 = call "iFlex - Prepare for Acquisition.vi"() -> ("Open iFlex Global Shutter"=w303:variant)  [unwired: 11 in]
        n215 = Send Notification(notification=w303, notifier=w311) -> (error out=w302:errorcluster)  [unwired: 1 in, 1 out]
        n216 = property on="Master Stop" class="Bool (strict)"("DisabledEnum"=w304) -> ()  [unwired: 2 in, 2 out]
        n217 = property on="Start Experiment" class="Bool"("DisabledEnum"=w304) -> ()  [unwired: 2 in, 2 out]
        n218 = global read "Global Controls.vi" "Tweezertron Ctrl Refs"() -> (w305:T13)
        n219 = property on="Exp Params" class="Clust (strict)"() -> ("Value"=w300:T9)  [unwired: 2 in, 2 out]
        n220 = call "Check if Folder exists.vi"("error in (no error)"=w302, "Exp Params in"=w300) -> ("error out"=w301:errorcluster, "Exp Params out"=w299:T9)  [unwired: 8 in]
        n221 = Unbundle By Name(w299) -> ("Experiment Type"=w306:string)
        n222 = To Variant(anything=w305) -> (Variant=w307:variant)
        n223 = Bundle("Experiment Type"=w306, "Variant"=w307) -> (w313:T22)  [unwired: 1 in]
        n224 = To Variant(anything=w313) -> (Variant=w314:variant)
        n225 = Send Notification(notification=w314, notifier=w309, error in (no error)=w301) -> ()  [unwired: 2 out]
        n226 = property on="Stop Experiment" class="Bool (strict)"("DisabledEnum"=T12."Enabled" ("Disabled")) -> ()  [unwired: 2 in, 2 out]
        n227 = property on="status" class="Str"("Value"="Running Experiment" ("status")) -> ()  [unwired: 2 in, 2 out]
      }
      event "Review Experiment": Value Change {
        w317 = T12."Disabled and Grayed Out" ("Disabled")
        n228 = event-data() -> ()  [unwired: 1 in, 1 out]
        n229 = Unbundle By Name(w322) -> ("Review Exp"=w323:refnum<notifier>)
        n230 = global read "Global Controls.vi" "Tweezertron Ctrl Refs"() -> (w320:T13)
        n231 = To Variant(anything=w320) -> (Variant=w319:variant)
        n232 = property on="Review Experiment" class="Bool (strict)"("Value"=FALSE ("Review Experiment")) -> ()  [unwired: 2 in, 2 out]
        n233 = property on="Review Experiment" class="Bool (strict)"("DisabledEnum"=w317) -> ()  [unwired: 2 in, 2 out]
        n234 = property on="Save TIFFs" class="Bool (strict)"("DisabledEnum"=w317) -> ()  [unwired: 2 in, 2 out]
        n235 = Bundle("Review Experiment", "Variant"=w319) -> (w324:cluster{string, "Variant":variant})  [unwired: 1 in]
        n236 = To Variant(anything=w324) -> (Variant=w325:variant)
        n237 = Send Notification(notification=w325, notifier=w323) -> ()  [unwired: 1 in, 2 out]
        n238 = property on="End Review" class="Bool (strict)"("DisabledEnum"=T12."Enabled" ("Disabled")) -> ()  [unwired: 2 in, 2 out]
        "Live Review" <- TRUE ("Live Imaging")
      }
      event "End Review": Value Change {
        n239 = event-data() -> ()  [unwired: 1 in, 1 out]
      }
      event "Save TIFFs": Value Change {
        w326 = T12."Disabled and Grayed Out" ("Disabled")
        n240 = event-data() -> ()  [unwired: 1 in, 1 out]
        n241 = Unbundle By Name(w331) -> ("Review Exp"=w332:refnum<notifier>)
        n242 = global read "Global Controls.vi" "Tweezertron Ctrl Refs"() -> (w329:T13)
        n243 = property on="Save TIFFs" class="Bool (strict)"("Value"=FALSE ("Review Experiment")) -> ()  [unwired: 2 in, 2 out]
        n244 = To Variant(anything=w329) -> (Variant=w328:variant)
        n245 = Bundle("Convert TDMS To TIFFs", "Variant"=w328) -> (w333:cluster{string, "Variant":variant})  [unwired: 1 in]
        n246 = property on="Save TIFFs" class="Bool (strict)"("DisabledEnum"=w326) -> ()  [unwired: 2 in, 2 out]
        n247 = property on="Review Experiment" class="Bool (strict)"("DisabledEnum"=w326) -> ()  [unwired: 2 in, 2 out]
        n248 = To Variant(anything=w333) -> (Variant=w334:variant)
        n249 = Send Notification(notification=w334, notifier=w332) -> ()  [unwired: 1 in, 2 out]
      }
      event Panel Close? {
        n250 = event-data() -> ()  [unwired: 1 in, 1 out]
        n251 = Two Button Dialog(message="Do you want to Exit?", 1:"No" ("F button name (\"Cancel\")"), 2:"Yes" ("T button name (\"OK\")")) -> (T button?=w335:bool)
        "pane closed" <- w335
        n252 = property on="Master Stop" class="Bool (strict)"("Val(Sgnl)"=w335) -> ()  [unwired: 2 in, 2 out]
        n253 = Not(x=w335) -> (.not. x?=w336:bool)
        n254 = event-data("Discard?"=w336) -> ()  [unwired: 1 in, 1 out]
      }
      event "Control Tabs": Value Change {
        n255 = event-data() -> ("NewVal"=w343:T2)  [unwired: 1 in]
        n256 = property on="Live Review" class="Bool (strict)"() -> ("Value"=w341:bool)  [unwired: 2 in, 2 out]
        n257 = property on="Live Imaging" class="Bool (strict)"() -> ("Value"=w346:bool)  [unwired: 2 in, 2 out]
        n258 = Not Equal?(x=w343, y=T2."System Controls" ("NewVal")) -> (x != y?=w347:bool)
        n259 = Not Equal?(x=T2."Review" ("NewVal"), y=w343) -> (x != y?=w342:bool)
        n260 = And(x=w347, y=w346) -> (x .and. y?=w345:bool)
        n261 = And(x=w341, y=w342) -> (x .and. y?=w340:bool)
        n262 = case shown="True" w340 {
          selector: w340 -> [_ w349]
          frame False {
          }
          frame True {
            n263 = property on="End Review" class="Bool (strict)"("Value"=w349) -> ()  [unwired: 2 in, 2 out]
          }
        }
        n264 = case shown="True" w345 {
          selector: w345 -> [_ w350]
          frame False {
          }
          frame True {
            n265 = property on="Stop Live Imaging" class="Bool (strict)"("Val(Sgnl)"=w350, "Value"=w350) -> ()  [unwired: 2 in, 2 out]
          }
        }
      }
      event "Master Stop": Value Change; Application Instance Close {
        n266 = event-data() -> ()  [unwired: 1 in, 1 out]
        n267 = global read "Global Controls.vi" "Tweezertron Ctrl Refs"() -> (w362:T13)
        n268 = Unbundle By Name(w363) -> ("Review Exp"=w352:refnum<notifier>, "LSM Run Exp"=w369:refnum<notifier>, "LSM Run Live"=w364:refnum<notifier>, "Instrument Control"=w366:refnum<notifier>)
        n269 = call <vilib>:"Application Directory.vi"() -> ("Application Directory"=w357:path)
        n270 = Release Notifier(notifier=w366) -> (error out=w367:errorcluster)  [unwired: 2 in, 2 out]
        n271 = Release Notifier(notifier=w364, error in (no error)=w367) -> (error out=w368:errorcluster)  [unwired: 1 in, 2 out]
        n272 = Release Notifier(notifier=w369, error in (no error)=w368) -> (error out=w370:errorcluster)  [unwired: 1 in, 2 out]
        n273 = Release Notifier(notifier=w352, error in (no error)=w370) -> (error out=w371:errorcluster)  [unwired: 1 in, 2 out]
        n274 = call "Write Settings XML.vi"("error in (no error)"=w371, "Tweezertron Ctrl Refs"=w362, "name or relative path"=".Last Session", "path"=w357) -> ("error out"=w361:errorcluster)  [unwired: 7 in]
        n275 = call "iFlex-Shutdown .vi"("error in"=w361) -> ("error out"=w360:errorcluster)  [unwired: 6 in]
        n276 = call "Teardown Device.vi"("error in (no error)"=w360) -> ("error out"=w359:errorcluster)  [unwired: 9 in, 1 out]
        n277 = property on="Manlight Controls" class="Clust (strict)"() -> ("Value"=w354:T4)  [unwired: 2 in, 2 out]
        n278 = Unbundle By Name(w354) -> ("VISA Refnum"=w353:refnum<visa-resource-name>)
        n279 = call "Teardown Camera.vi"("error in (no error)"=w359) -> ("error out"=w358:errorcluster)  [unwired: 5 in, 1 out]
        n280 = call "Teardown Device.vi"("error in (no error)"=w358) -> ("error out"=w356:errorcluster)  [unwired: 5 in, 1 out]
        n281 = call "Manlight-Connection.vi"("error in"=w356, "Connect?"=FALSE, "VISA Refnum in"=w353) -> ("error out"=w351:errorcluster)  [unwired: 1 in, 3 out]
        n282 = call "Close Hologram Engine.vi"("error in (no error)"=w351) -> ()  [unwired: 11 in]
      }
    }
  }
  n283 = while {
    tunnel: w3 -> [w377]
    stop <- w375 stop-if-true
    # "Instrument Control - SLAVE"
    n284 = call "Receive and Prepare Messages.vi"("Notifiers"=w377) -> ("error out"=w376:errorcluster, "params"=w374:variant, "message"=w373:string)  [unwired: 8 in]
    n285 = case shown="No Error" w376 {
      selector: w376 -> [w379 w404]
      tunnel: w373 -> [w381 _]
      tunnel: w374 -> [w380 _]
      tunnel: [w378 w404] -> w375
      frame No Error {
        n286 = case shown="\"Update SLM\"" w381 {
          tunnel: w380 -> [_ w386 w389 w391 w395 w398 _ w401]
          tunnel: w379 -> [w382 w385 w388 w392 _ w399 w400 w402]
          tunnel: [w382 w384 w387 w390 _ w397 w400 w403] -> w378
          frame Default {
          }
          frame "Update LSM" {
            # "LSM Setting"
            n287 = call "Thorlabs-Update Settings.vi"("error in (no error)"=w385, "params"=w386) -> ("error out"=w384:errorcluster, "Pause Live Imaging"=w383:bool)  [unwired: 8 in]
            n288 = local write "Pause Live Imaging"(w383) -> ()
          }
          frame "Update Pin" {
            n289 = call "Thorlabs-Update Pinhole.vi"("error in (no error)"=w388, "params"=w389) -> ("error out"=w387:errorcluster)  [unwired: 9 in]
          }
          frame "Update SLM" {
            n290 = call "Update UDP.vi"("error in (no error)"=w392, "params"=w391) -> ("error out"=w390:errorcluster)  [unwired: 9 in]
          }
          frame "Update Manlight" {
            n291 = property on="Manlight Controls" class="Clust (strict)"() -> ("Value"=w394:T4)  [unwired: 2 in, 2 out]
            n292 = Unbundle By Name(w394) -> ("VISA Refnum"=w393:refnum<visa-resource-name>)
            n293 = call "Manlight - Update Power.vi"("VISA resource name"=w393, "params"=w395) -> ()  [unwired: 4 in, 2 out]
          }
          frame "Update PIFOC" {
            # "PIFOC Settings"
            n294 = call "PI-Move PIFOC.vi"("error in (no error)"=w399, "params"=w398) -> ("error out"=w397:errorcluster, "PIFOC out"=w396:T6)  [unwired: 8 in]
            n295 = property on="PIFOC Settings" class="Clust (strict)"("Value"=w396) -> ()  [unwired: 2 in, 2 out]
          }
          frame "Update MCSL" {
            # "MCSL Settings"
          }
          frame "Update iFlex" {
            n296 = call "iFlex 2.0 .vi"("error in"=w402, "params"=w401) -> ("error out"=w403:errorcluster)  [unwired: 9 in]
          }
        }
      }
      frame Error {
      }
    }
  }
  n297 = while {
    tunnel: w3 -> [w410]
    tunnel: w2 -> [w406]
    stop <- w409 stop-if-true
    # "Aquiring Data"
    n298 = call "Receive and Prepare Messages Run.vi"("Notifiers"=w410) -> ("error out"=w405:errorcluster, "params"=w407:variant, "message"=w408:string)  [unwired: 7 in]
    n299 = case shown="No Error" w405 {
      selector: w405 -> [w420 w530]
      tunnel: [w418 w530] -> w409
      tunnel: w408 -> [w433 _]
      tunnel: w407 -> [w427 _]
      tunnel: w406 -> [w425 w529]
      frame No Error {
        n300 = Variant To Data(error in=w420, type=T13 {"LSM Settings"=refnum, "iFlex Control"=refnum, "PIFOC Settings"=refnum, "PinSelector"=refnum, "Manlight Controls"=refnum, "Exp Params"=refnum, "Image Thresholds"=refnum, "RevFrame"=refnum, "Spots"=refnum} ("Tweezertron Ctrl Refs"), Variant=w427) -> (data=w413:T13, error out=w429:errorcluster)
        n301 = Unbundle By Name(w413) -> ("Exp Params"=w430:refnum<vi>)
        n302 = property class="Clust (strict)"(reference=w430) -> ("Value"=w423:T9)  [unwired: 1 in, 2 out]
        n303 = Unbundle By Name(w413) -> ("PIFOC Settings"=w432:refnum<vi>)
        n304 = property class="Clust (strict)"(reference=w432) -> ("Value"=w417:T6)  [unwired: 1 in, 2 out]
        n305 = call "Prepare Logging Loop.vi"("error in (no error)"=w429, "Tweezertron Ctrl Refs"=w413, "Queue in"=w425) -> ("error out"=w416:errorcluster, "Tweezertron Ctrl Refs out"=w412:T13, "Queue out"=w421:refnum<queue>)  [unwired: 6 in]
        n306 = global read "Global1.vi" "DLL device ID's"() -> (w431:i32[])
        n307 = control-ref of="Acquiring Data"() -> (w422:refnum<vi>)
        n308 = call "Thorlabs-Start Scanning.vi"("error in (no error)"=w416, "Tweezertron Ctrl Refs"=w412) -> ("error out"=w415:errorcluster, "Tweezertron Ctrl Refs out"=w411:T13, "pDataBuffer"=w414:u16[])  [unwired: 7 in]
        n309 = Index Array(array=w431, index=0) -> (element=w424:i32)
        n310 = case shown="\"3D Snapshot\"" w433 {
          tunnel: w415 -> [w443 w454 w497 w519]
          tunnel: [w450 w461 w494 w520] -> w435
          tunnel: w421 -> [w452 w463 w504 w522]
          tunnel: [w451 w462 w503 w521] -> w438
          tunnel: w422 -> [_ w460 w493 w513]
          tunnel: w423 -> [_ w459 w501 w509]
          tunnel: w424 -> [_ _ w498 w515]
          tunnel: w417 -> [w445 w456 _ _]
          tunnel: w414 -> [w442 w453 w490 w511]
          frame "2D Snapshot", Default {
            # "1. Start Scanner\n2. Get PIFOC Pos ACT\n3. Get system time in seconds\n4. Get pData from PMTs\n5. Send for processing"
            n311 = Unbundle By Name(w445) -> ("PIFOC Position\n(um) [ACT]"=w444:dbl)
            n312 = Get Date/Time In Seconds() -> (seconds since 1Jan1904=w447:timestamp)
            n313 = To Unsigned Quad Integer(1:w447) -> (0:w446:u64)
            n314 = call "Thorlabs-Acquire Next Image.vi"("error in (no error)"=w443, "pDataBuffer in"=w442) -> ("error out"=w449:errorcluster, "pDataBuffer out"=w448:u16[])  [unwired: 7 in, 1 out]
            n315 = call "Que Data To Process.vi"("queue in"=w452, "error in (no error)"=w449, "PIFOC Pos"=w444, "timestamp (nm)"=w446, "pDataBuffer in"=w448) -> ("error out"=w450:errorcluster, "queue out"=w451:refnum<queue>)  [unwired: 5 in]
          }
          frame "2D Time Series" {
            # "1. Start Scanners\n2. Get PIFOC Pos ACT\n3. While have frames\n   a. Get pData from PMT\n   b. Get iteration start time\n   c. Send for processing"
            n316 = Unbundle By Name(w459) -> ("period"=w458:i32, "total images"=w457:i32)
            n317 = Unbundle By Name(w456) -> ("PIFOC Position\n(um) [ACT]"=w455:dbl)
            n318 = To Quad Integer(1:w458) -> (0:w464:i64)
            n319 = node-c288(w464) -> (w466:T23)
            n320 = timed-loop {
              tunnel: w454 -> [w481]
              timing: w466 -> [_]
              timing-out: [_] -> w465
              tunnel: w453 -> [w479]
              tunnel: w457 -> [w478]
              tunnel: w463 -> [w475]
              tunnel: [w474] -> w462
              tunnel: [w477] -> w461
              tunnel: w460 -> [w473]
              tunnel: w455 -> [w468]
              i -> [w472]
              stop <- w471 stop-if-true
              n321 = node-c288() -> (w467:i64)  [unwired: 1 in]
              n322 = call "Thorlabs-Acquire Next Image.vi"("error in (no error)"=w481, "pDataBuffer in"=w479) -> ("error out"=w470:errorcluster, "pDataBuffer out"=w476:u16[])  [unwired: 7 in, 1 out]
              n323 = global read "Global Controls.vi" "Stop Experiment"() -> (w469:bool)
              n324 = Equal?(x=w478, y=w472) -> (x = y?=w480:bool)
              n325 = property class="Slide (strict)"(reference=w473, "Value"=w472) -> ()  [unwired: 1 in, 2 out]
              n326 = call "Que Data To Process.vi"("queue in"=w475, "error in (no error)"=w470, "PIFOC Pos"=w468, "timestamp (nm)"=w467, "pDataBuffer in"=w476) -> ("error out"=w477:errorcluster, "queue out"=w474:refnum<queue>)  [unwired: 5 in]
              n327 = Or(x=w469, y=w480) -> (x .or. y?=w471:bool)
            }
            n328 = node-c288(w465) -> ()
          }
          frame "3D Snapshot" {
            # "1. Move Pifoc to start position\n2. Start Scanners\n3. Pause for scanners to start\n4. Aquire single stack\n5. Move Pifoc back to start"
            n329 = Unbundle By Name(w501) -> ("Z Stack Settings.Start"=w500:dbl, "images per stack"=w495:i32, "PI MVR Increment"=w489:string)
            n330 = call "PI-Double To String.vi"("Start"=w500, "String in"="MOV") -> ("String out"=w492:string)  [unwired: 2 in]
            n331 = call "PI MVR.vi"("error in (no error)"=w497, "String"=w492, "PI ID in"=w498) -> ("error out"=w491:errorcluster, "PI ID out"=w496:i32)  [unwired: 6 in, 1 out]
            n332 = flat-sequence {
              tunnel: [w508] -> w499
              tunnel: w491 -> [w508]
              frame #0 {
                n333 = Wait (ms)(milliseconds to wait=u32 200) -> ()  [unwired: 1 out]
              }
            }
            n334 = call "Aquire Z-Stack.vi"("Acquisition Progres Bar"=w493, "Move Relative Increment"=w489, "queue in"=w504, "error in (no error)"=w499, "Number of slices"=w495, "PI ID in"=w496, "pDataBuffer"=w490) -> ("error out"=w505:errorcluster, "PI ID out"=w502:i32, "queue out"=w503:refnum<queue>)  [unwired: 2 in]
            n335 = call "PI MVR.vi"("error in (no error)"=w505, "String"=w492, "PI ID in"=w502) -> ("error out"=w494:errorcluster)  [unwired: 6 in, 2 out]
          }
          frame "3D Time Series" {
            n336 = Unbundle By Name(w509) -> ("Z Stack Settings.Start"=w517:dbl)
            n337 = control-ref of="#stack"() -> (w523:refnum<vi>)
            n338 = call "PI-Double To String.vi"("Start"=w517, "String in"="MOV") -> ("String out"=w516:string)  [unwired: 2 in]
            n339 = call "PI MVR.vi"("error in (no error)"=w519, "String"=w516, "PI ID in"=w515) -> ("error out"=w512:errorcluster, "PI ID out"=w510:i32)  [unwired: 6 in, 1 out]
            n340 = flat-sequence {
              tunnel: [w525] -> w514
              tunnel: w512 -> [w525]
              frame #0 {
                n341 = Wait (ms)(milliseconds to wait=u32 200) -> ()  [unwired: 1 out]
              }
            }
            n342 = call "Aquire Multi Z-Stack.vi"("#stack"=w523, "Acquisition Progres Bar"=w513, "queue in"=w522, "error in (no error)"=w514, "Exp Params"=w509, "PI ID"=w510, "pDataBuffer"=w511) -> ("error out"=w520:errorcluster, "queue out"=w521:refnum<queue>)  [unwired: 3 in]
          }
        }
        n343 = property on="status" class="Str"(error in=w435, "Value"="Finished Aquiring data. Saving to disk" ("status")) -> (error out=w434:errorcluster)  [unwired: 1 in, 1 out]
        n344 = call "Que Close TDMS.vi"("error in (no error)"=w434, "Tweezertron Ctrl Refs"=w411, "Queue in"=w438) -> ("error out"=w437:errorcluster)  [unwired: 8 in]
        n345 = call "Thorlabs-Stop.vi"("error in (no error)"=w437) -> ("error out"=w419:errorcluster)  [unwired: 10 in]
        n346 = flat-sequence {
          tunnel: w419 -> [w441]
          tunnel: [w441] -> w418
          frame #0 {
            w440 = T12."Enabled" ("Disabled")
            n347 = property on="Master Stop" class="Bool (strict)"("DisabledEnum"=w440) -> ()  [unwired: 2 in, 2 out]
            n348 = property on="Start Experiment" class="Bool"("DisabledEnum"=w440) -> ()  [unwired: 2 in, 2 out]
            n349 = property on="Stop Experiment" class="Bool (strict)"("DisabledEnum"=T12."Disabled and Grayed Out" ("Disabled")) -> ()  [unwired: 2 in, 2 out]
          }
        }
      }
      frame Error {
        # "This will error when the Notifs are killed. So now we can stop the logging loop"
        n350 = Bundle By Name(cluster=T26 {"message"="", "Data for Logging"={"pDataBuffer"=[], "timestamp (ns)"=0, "PI pos (um)"=0.0}, "Tweezertron Ctrl Refs"={"LSM Settings"=refnum, "iFlex Control"=refnum, "PIFOC Settings"=refnum, "PinSelector"=refnum, "Manlight Controls"=refnum, "Exp Params"=refnum, "Image Thresholds"=refnum, "RevFrame"=refnum, "Spots"=refnum}} ("Logging Queue Cluster"), "message"="Stop") -> (w526:T26)
        n351 = Enqueue Element(queue=w529, element=w526) -> ()  [unwired: 2 in, 3 out]
      }
    }
  }
  n352 = while {
    tunnel: w2 -> [w534]
    shift-right: [w537] -> _
    shift-left: _ -> [w538]
    stop <- w531 stop-if-true
    # "Processing Data"
    n353 = Dequeue Element(queue=w534) -> (queue out=w532:refnum<queue>, element=w535:T26, error out=w533:errorcluster)  [unwired: 2 in, 1 out]
    n354 = Unbundle By Name(w535) -> ("message"=w536:string)
    n355 = case shown="No Error" w533 {
      selector: w533 -> [w544 _]
      tunnel: w536 -> [w545 _]
      tunnel: w538 -> [w543 w570]
      tunnel: [w542 w570] -> w537
      tunnel: w535 -> [w541 _]
      tunnel: w532 -> [w540 _]
      tunnel: [w539 TRUE] -> w531
      frame No Error {
        n356 = case shown="\"Save TDMS\"" w545 {
          tunnel: w544 -> [_ w558 w564 w567]
          tunnel: w543 -> [_ w557 w563 w568]
          tunnel: [w549 w552 w563 w568] -> w542
          tunnel: w541 -> [w548 w556 w561 _]
          tunnel: w540 -> [_ _ w562 w566]
          tunnel: [_ _ _ TRUE] -> w539
          frame "Push All Params", Default {
            n357 = Unbundle By Name(w548) -> ("Tweezertron Ctrl Refs.Exp Params"=w547:refnum<vi>)
            n358 = property class="Clust (strict)"(reference=w547) -> ("Value"=w546:T9)  [unwired: 1 in, 2 out]
            n359 = Bundle By Name(cluster=w546, "frame #"=i64 0) -> (w549:T9)
          }
          frame "Save TDMS" {
            n360 = Unbundle By Name(w556) -> ("Data for Logging.pDataBuffer"=w555:u16[], "Data for Logging.timestamp (ns)"=w554:u64, "Data for Logging.PI pos (um)"=w553:dbl)
            n361 = call "Save to TDMS.vi"("Exp Params in"=w557, "error in (no error)"=w558, "PI pos (um)"=w553, "Timestamps (ns)"=w554, "pDataBuffer"=w555) -> ("Exp Params in out"=w552:T9)  [unwired: 5 in, 1 out]
            n362 = Unbundle By Name(w552) -> ("frame #"=w551:i64)
            n363 = property on="Saving To Disk" class="Slide (strict)"("Value"=w551) -> ()  [unwired: 2 in, 2 out]
          }
          frame "Close TDMS" {
            n364 = call "Close TDMS and Save XML.vi"("error in (no error)"=w564, "Logging Queue Cluster"=w561, "Exp Params in in"=w563, "Queue in"=w562) -> ("Review Path"=w559:path)  [unwired: 7 in]
            n365 = property on="Rev Path" class="Path"("Value"=w559) -> ()  [unwired: 2 in, 2 out]
            n366 = property on="status" class="Str"("Value"="Ready" ("status")) -> ()  [unwired: 2 in, 2 out]
          }
          frame "Stop" {
            n367 = Release Queue(queue=w566, error in (no error)=w567) -> ()  [unwired: 1 in, 3 out]
          }
        }
      }
      frame Error {
      }
    }
  }
  n368 = while {
    tunnel: w3 -> [w575]
    stop <- w576 stop-if-true
    # "Review Data"
    n369 = call "Receive and Prepare Messages Review.vi"("Notifiers"=w575) -> ("error out"=w573:errorcluster, "params"=w572:variant, "message"=w574:string, "Review Exp"=w571:refnum<notifier>)  [unwired: 6 in]
    n370 = case shown="No Error" w573 {
      selector: w573 -> [w580 w678]
      tunnel: w574 -> [w581 _]
      tunnel: [_ w678] -> w576
      tunnel: w572 -> [w578 _]
      tunnel: w571 -> [w579 _]
      frame No Error {
        n371 = case shown="\"Review Experiment\", Default" w581 {
          tunnel: w580 -> [_ _ w664 w674]
          tunnel: w579 -> [w589 w620 _ _]
          tunnel: w578 -> [_ _ w665 w675]
          tunnel: "Rev Path" -> [w584 w622 _ _]
          frame "Review Experiment", Default {
            n372 = call "Open TDMS.vi"("RevPath"=w584) -> ("TDMS File Found"=w585:bool, "RevPath out"=w586:path, "tdms file out"=w587:refnum<k34>)  [unwired: 8 in]
            n373 = call "Get SettingsXML from Path.vi"("TDMS File Found"=w585, "Rev Path"=w586, "tdms file in"=w587) -> ("XML File Found"=w583:bool, "tdms file out"=w588:refnum<k34>)  [unwired: 5 in, 2 out]
            n374 = case shown="True" w583 {
              tunnel: w588 -> [w590 w594]
              tunnel: [w590 w592] -> w582
              frame False {
              }
              frame True {
                w604 = T10 6 items=["Grayscale (U8)", "Grayscale (I16)", "Grayscale (SGL)", "Complex (CSG)", "RGB (U32)", "HSL (U32)", "RGB (U64)", "Grayscale (U16)"] ("Image Type")
                n375 = call "Read in TDMS.vi"("tdms in"=w594) -> ("PI pos (um)"=w595:dbl[], "Timestamps (ms)"=w596:u64[], "tdms file out"=w597:refnum<k34>)  [unwired: 7 in, 1 out]
                n376 = call "Prepare Data for Review.vi"("PI pos (um)"=w595, "Timestamps (ms)"=w596) -> ("PI pos (um) out"=w599:dbl[], "dts"=w598:u64[], "Time (s)"=w593:dbl[], "PIFOC Graph"=→"PIFOC Positions":cluster{dbl[], "PI pos (um)":dbl[]})  [unwired: 6 in]
                "dts (ms)" <- w598
                n377 = call "IMAQ Create"("Image Name"="Rev RGB", "Image Type"=w604) -> ("New Image"=w602:T1)  [unwired: 3 in, 1 out]
                n378 = while {
                  shift-right: [w606] -> w601
                  shift-left: w602 -> [w617]
                  shift-right: [w614] -> w592
                  shift-left: w597 -> [w616]
                  tunnel: w593 -> [w610]
                  tunnel: w598 -> [w609]
                  tunnel: w599 -> [w608]
                  stop <- "End Review" stop-if-true
                  n379 = call "Read Frame From TDMS.vi"("Frame Number"="RevFrame", "tdms file in"=w616) -> ("tdms file out"=w614:refnum<k34>, "pDataBuffer"=w615:u16[])  [unwired: 7 in, 1 out]
                  n380 = call "pDataBufferToRGBimage.vi"("Img Dst"=w617, "pDataBuffer"=w615) -> ("Img Out"=w606:refnum<image>)  [unwired: 8 in, 1 out]
                  n381 = call "Select Review Frame.vi"("RevFrame"="RevFrame", "PI pos (um) in"=w608, "dts"=w609, "Time (s) in"=w610) -> ("Position (um)"=→"Position (um)":dbl, "dt (ms)"=→"dt (ms)":u32, "Time (s) out"=→"Time (s)":dbl)  [unwired: 5 in]
                  n382 = property on="status" class="Str"("Value"="Reviewing Experiment" ("status")) -> ()  [unwired: 2 in, 2 out]
                  n383 = property on="LiveDisp" class="ImageControl"("Value"=w606) -> ()  [unwired: 2 in, 2 out]
                }
                n384 = call "IMAQ Dispose"("Image"=w601) -> ()  [unwired: 5 in, 1 out]
                n385 = property on="status" class="Str"("Value"="Loading Experiemnt. This can take a few minutes for large experiments and cannot be aborted until loading is finished." ("status")) -> ()  [unwired: 2 in, 2 out]
              }
            }
            n386 = call "Closing Sequence For Review.vi"("tdms file"=w582, "Notifier in"=w589) -> ()  [unwired: 10 in]
          }
          frame "Convert TDMS To TIFFs" {
            n387 = call "Open TDMS.vi"("RevPath"=w622) -> ("TDMS File Found"=w623:bool, "RevPath out"=w624:path, "tdms file out"=w625:refnum<k34>)  [unwired: 8 in]
            n388 = call "Get SettingsXML from Path.vi"("TDMS File Found"=w623, "Rev Path"=w624, "tdms file in"=w625) -> ("XML File Found"=w619:bool, "Controls"=w626:T15, "Rev Path out"=w627:path, "tdms file out"=w628:refnum<k34>)  [unwired: 5 in]
            n389 = case shown="True" w619 {
              tunnel: w628 -> [w629 w638]
              tunnel: w627 -> [_ w637]
              tunnel: w626 -> [_ w636]
              tunnel: [w629 w631] -> w621
              frame False {
              }
              frame True {
                n390 = Unbundle By Name(w636) -> ("Exp Params.total images"=w630:i32, "Confocal Controls"=w646:T5, "Confocal Controls.Channel Selection"=w645:enum32{"A", "B", "AB"})
                n391 = call "Read in TDMS.vi"("tdms in"=w638) -> ("PI pos (um)"=w639:dbl[], "Timestamps (ms)"=w640:u64[], "tdms file out"=w641:refnum<k34>)  [unwired: 7 in, 1 out]
                n392 = call "Create TIFFs Folder.vi"("Rev Path"=w637) -> ("Path To Exp"=w632:path, "Path to TIFFS"=w643:path)  [unwired: 9 in]
                n393 = call "Save PIFOC to TXT.vi"("Path To Exp"=w632, "PI pos (um)"=w639) -> ("Path To Exp out"=w633:path)  [unwired: 9 in]
                n394 = call "Save Timestamps to TXT.vi"("Path To Exp"=w633, "Timestamps (ms)"=w640) -> ()  [unwired: 9 in, 1 out]
                n395 = property on="status" class="Str"("Value"="Exporting TIFFs" ("status")) -> ()  [unwired: 2 in, 2 out]
                n396 = property on="Exporting TIFFS" class="Slide (strict)"("Scale.Maximum"=w630) -> ()  [unwired: 2 in, 2 out]
                n397 = call "Convert Channel Selection To String.vi"("Channel Selection"=w645) -> ("Channel Name(s)"=w644:string[])  [unwired: 4 in]
                n398 = call "Create IMAQ Img from Channels.vi"("Channel Name(s)"=w644) -> ("IMAQ Ch Images"=w634:T1[], "Channel Name(s) out"=w635:string[])  [unwired: 3 in]
                n399 = for {
                  N: w630 -> [_]
                  tunnel: [w653] -> w647
                  tunnel: w646 -> [w652]
                  tunnel: w634 -> [w657]
                  tunnel: w635 -> [w656]
                  tunnel: w643 -> [w655]
                  shift-right: [w651] -> w631
                  shift-left: w641 -> [w659]
                  i -> [w649]
                  n400 = Increment(x=w649) -> (x+1=w650:i32)
                  n401 = call "Get Frame from TDMS.vi"("Channel Name(s)"=w656, "Frame Number"=w649, "base path"=w655, "TDMS Ref"=w659) -> ("Paths for TIFFs"=w654:path[], "tdms file out"=w651:refnum<k34>, "pDataBuffer"=w658:u16[])  [unwired: 5 in]
                  n402 = property on="Exporting TIFFS" class="Slide (strict)"("Value"=w650) -> ()  [unwired: 2 in, 2 out]
                  n403 = call "Convert pData to TIFF.vi"("Img Dst Array"=w657, "pDataBuffer"=w658, "Paths for TIFFs"=w654, "Confocal Controls"=w652) -> ("Img Dst Array out"=w653:T1[])  [unwired: 7 in]
                }
                n404 = for {
                  tunnel: w647 -> [w648] mode=indexing
                  n405 = call "IMAQ Dispose"("Image"=w648) -> ()  [unwired: 5 in, 1 out]
                }
              }
            }
            n406 = call "Closing Sequence For Export TIFFs.vi"("tdms file"=w621, "Notifier in"=w620) -> ()  [unwired: 10 in]
          }
          frame "End Review" {
            w668 = FALSE ("End Review")
            w666 = T12."Enabled" ("Disabled")
            # "If we dont find a TDMS we still call this case so as to sort out the enabled ctrls.\nIn this case the Close TDMS errors so just clear it"
            n407 = Variant To Data(error in=w664, type=refnum<k34> refnum ("data"), Variant=w665) -> (data=w662:refnum<k34>, error out=w663:errorcluster)
            n408 = TDMS Close(8:w663, 11:w662) -> (0:w660:errorcluster)  [unwired: 1 out]
            n409 = call <vilib>:"Clear Errors.vi"("error in (no error)"=w660) -> ()  [unwired: 5 in, 2 out]
            n410 = property on="Save TIFFs" class="Bool (strict)"("DisabledEnum"=w666) -> ()  [unwired: 2 in, 2 out]
            n411 = property on="Review Experiment" class="Bool (strict)"("DisabledEnum"=w666) -> ()  [unwired: 2 in, 2 out]
            n412 = property on="End Review" class="Bool (strict)"("DisabledEnum"=T12."Disabled and Grayed Out" ("Disabled"), "Value"=w668) -> ()  [unwired: 2 in, 2 out]
            n413 = property on="Live Review" class="Bool (strict)"("Value"=w668) -> ()  [unwired: 2 in, 2 out]
            n414 = property on="status" class="Str"("Value"="Ready" ("status")) -> ()  [unwired: 2 in, 2 out]
          }
          frame "Finish Export" {
            w676 = T12."Enabled" ("Disabled")
            # "If we dont find a TDMS we still call this case so as to sort out the enabled ctrls.\nIn this case the Close TDMS errors so just clear it"
            n415 = Variant To Data(error in=w674, type=refnum<k34> refnum ("data"), Variant=w675) -> (data=w673:refnum<k34>, error out=w672:errorcluster)
            n416 = TDMS Close(8:w672, 11:w673) -> (0:w670:errorcluster)  [unwired: 1 out]
            n417 = property on="Save TIFFs" class="Bool (strict)"("DisabledEnum"=w676) -> ()  [unwired: 2 in, 2 out]
            n418 = property on="Review Experiment" class="Bool (strict)"("DisabledEnum"=w676) -> ()  [unwired: 2 in, 2 out]
            n419 = call <vilib>:"Clear Errors.vi"("error in (no error)"=w670) -> ()  [unwired: 5 in, 2 out]
            n420 = property on="status" class="Str"("Value"="Ready" ("status")) -> ()  [unwired: 2 in, 2 out]
          }
        }
      }
      frame Error {
      }
    }
  }
